vi "Do_ADAM_channel.vi"(4 "Scan Period":dbl format="%.2f", 5 "Previous Scan Value":dbl format="%.2f", 6 "Present scan array":dbl[](array[numeric]) format="%.2f", 7 "Value to Output":dbl format="%.2f", 8 "Ch Description":T1 {"Duty" format="%016b"; "D" format="%#_5g"; "C" format="%#_5g"; "B" format="%#_5g"; "A" format="%#_5g"}, 9 "Ch names":string[](array[string])) -> (0 "Scan comment":string, 1 "Output":dbl format="%.3f")   [LabVIEW 2016]
uses:
  ADAM Client/Sub VIs/ADAM Controls/Ch_description_ADAM.ctl
  ADAM Client/Sub VIs/ADAM Controls/Module_type_ADAM.ctl
  ADAM Client/Sub VIs/ADAM Controls/Function_ADAM.ctl
  ADAM Client/Sub VIs/ADAM Controls/Channel_State.ctl
  ADAM Client/Sub VIs/ADAM Controls/Calib_type_ADAM.ctl
  ADAM Client/Sub VIs/ADAM Controls/Address.ctl
  ADAM Client/Sub VIs/ADAM Controls/Remember_value_mode.ctl
  ADAM Serial/Instrument drivers/Arduino/ctls_and_globals/Arduino tx msg cluster.ctl
  <vilib>/Utility/error.llb/DialogType.ctl
  Anemometry/Anemometry Sub Vis/Controls/In_Range.ctl
  <vilib>/Analysis/baseanly.llb/Mean (DBL).vi
  ADAM Serial/Instrument drivers/LabJack/T7/T7Examples/MODBUS/T7MOD_Read_UINT16_Register.vi
  ADAM Serial/Instrument drivers/LabJack/T7/T7Examples/MODBUS/T7MOD_Read_UINT32_Register.vi
  ADAM Serial/Instrument drivers/LabJack/T7/T7Examples/MODBUS/T7MOD_Read_INT32_Register.vi
  ADAM Serial/Instrument drivers/LabJack/T7/T7Examples/MODBUS/T7MOD_Read_FLOAT32_Register.vi
  ADAM Serial/Instrument drivers/LabJack/T7/T7Examples/MODBUS/T7MOD_Write_UINT16_Register.vi
  ADAM Serial/Instrument drivers/LabJack/T7/T7Examples/MODBUS/T7MOD_Write_UINT32_Register.vi
  ADAM Serial/Instrument drivers/LabJack/T7/T7Examples/MODBUS/T7MOD_Write_INT32_Register.vi
  ADAM Serial/Instrument drivers/LabJack/T7/T7Examples/MODBUS/T7MOD_Write_FLOAT32_Register.vi
  Anemometry/Anemometry Sub Vis/Globals/Gas_management_global.vi
  ADAM_Global.vi
  Anemometry/Anemometry Sub Vis/Globals/Constants_global.vi
  <vilib>/Analysis/NI_AALBase.lvlib
panel:
  in  "MaxAge(s)":dbl=1.5
  in  "History Length":i32=150
  in  "K_Uni_chilled water":dbl=17.0
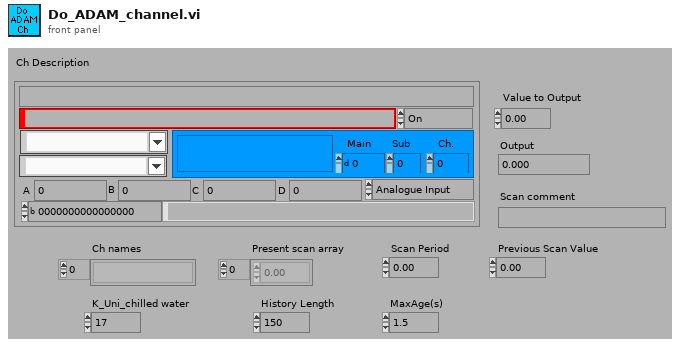
[diagram p1: front panel]
types:
  T1 = typedef "Ch_description_ADAM.ctl" = cluster{"Ch Name":string, "Type":T2, "Function":T3, "Ch State":T4, "Calibration type":T5, "A":dbl, "B":dbl, "C":dbl, "D":dbl, "Comments":string, "Address":T6, "String":string, "Duty":u16}
  T2 = typedef "Module_type_ADAM.ctl" = string
  T3 = typedef "Function_ADAM.ctl" = enum16{"Analogue Input", "Digital Input", "Event counter", "Event rate", "Analogue Output", "Digital Output", "Relay Output"}
  T4 = typedef "Channel_State.ctl" = enum16{"On", "Off", "Always On", "Always Off"}
  T5 = typedef "Calib_type_ADAM.ctl" = string
  T6 = typedef "Address.ctl" = cluster{"Main":i32, "Ch.":i32, "Sub":i32, "Port Name":string}
  T7 = typedef "Remember_value_mode.ctl" = enum16{"Read only", "Read and Write"}
  T8 = cluster{"error out":errorcluster, "source out":string, "message":string, "Read At":timestamp, dbl}
  T9 = cluster{"error out":errorcluster, "source out":string, "message":string}
  T10 = typedef "In_Range.ctl" = enum16{"%", "±", "% & ±"}
  T11 = typedef "Arduino tx msg cluster.ctl" = cluster{"dest":u8, "A/D/C/I":string, "R/W":string, "chan":u8, "val (float)":sgl}
  T12 = typedef "DialogType.ctl" = u16
  T13 = typedef "Valco_valve_ph.ctl" = u16
  T14 = typedef "LVDateTimeRec.ctl" = cluster{"fractional second":dbl, "second":i32, "minute":i32, "hour":i32, "day of month":i32, "month":i32, "year":i32, "day of week":i32, "day of year":i32, "DST":i32}
  T15 = typedef "Client_State_Cluster.ctl" = cluster{"Client Name":string, "Traverse level State":T16, "People to Email":string[], "Next Contact Time":dbl}
  T16 = typedef "Traverse_Level_State.ctl" = enum16{"Running", "Complete"}
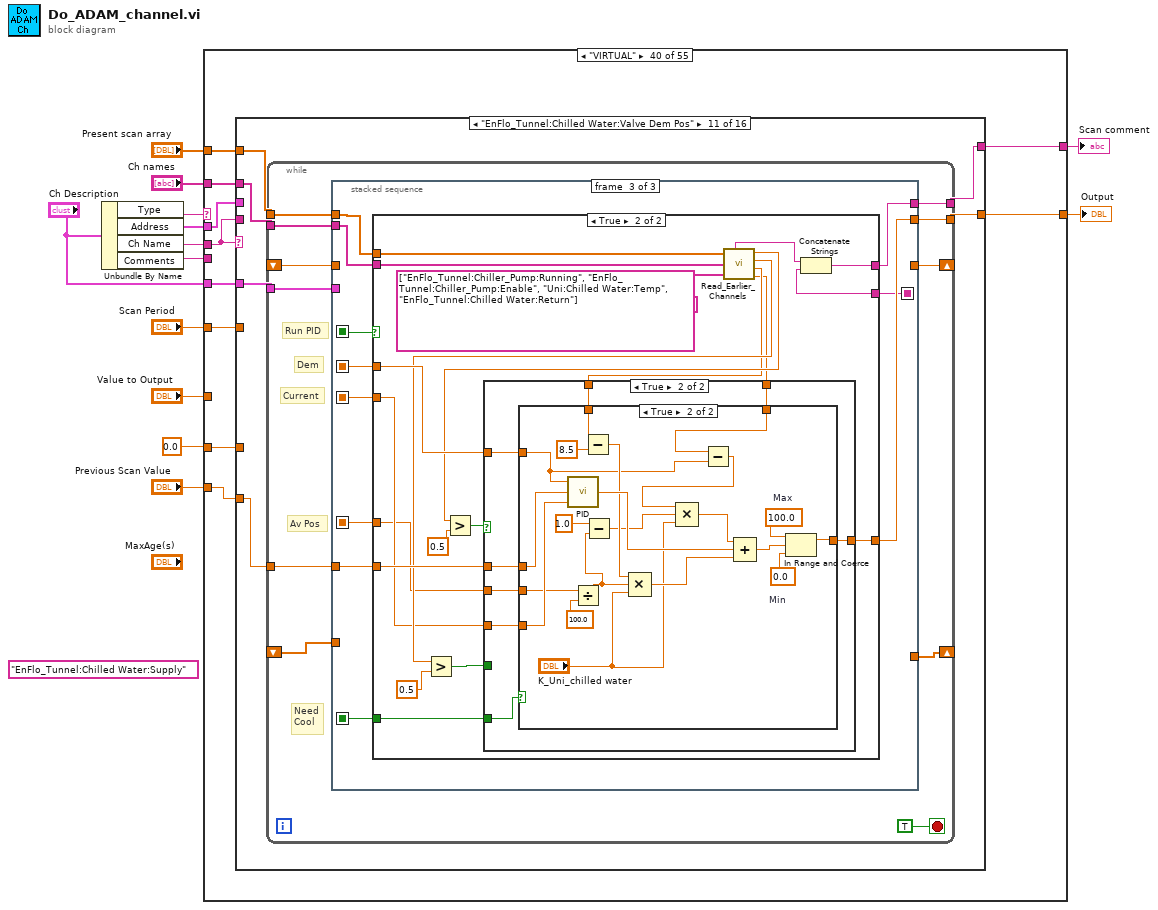
[diagram p0: block diagram]
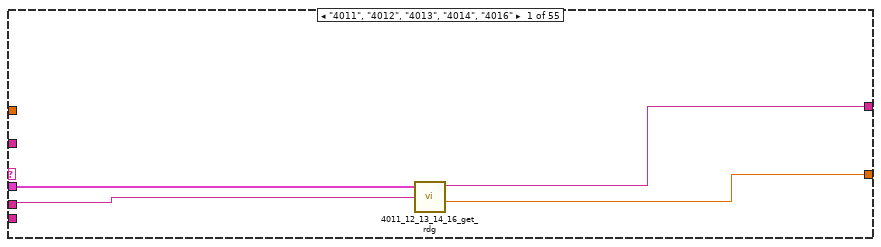
[diagram p2: hidden frame]
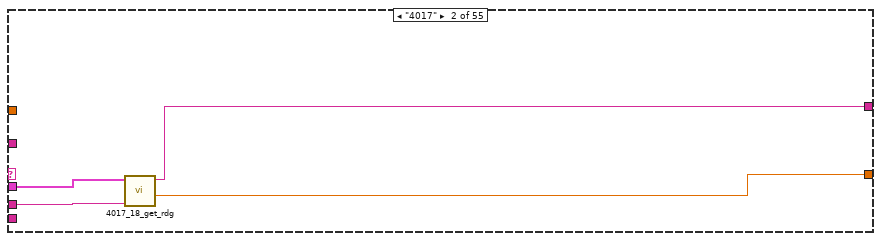
[diagram p3: hidden frame]
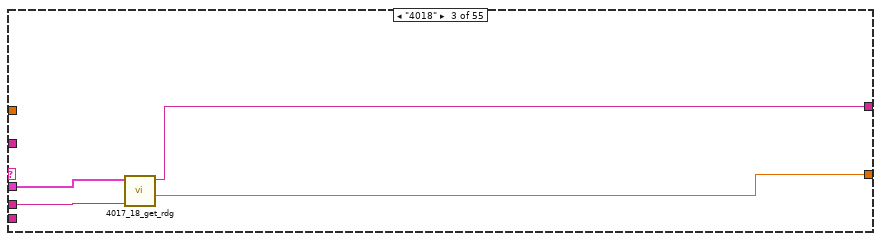
[diagram p4: hidden frame]
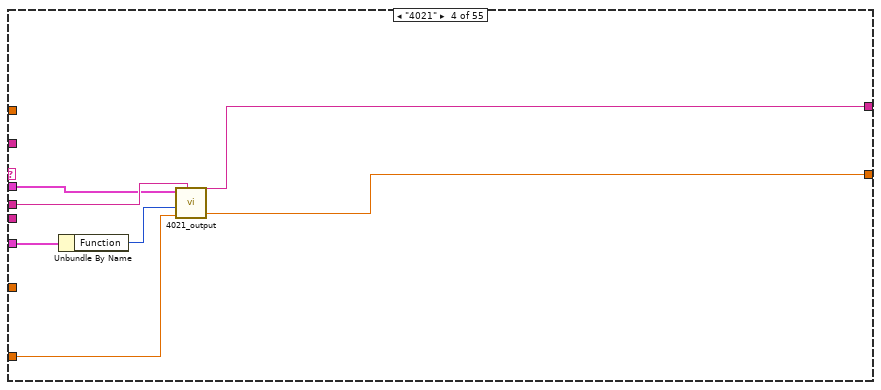
[diagram p5: hidden frame]
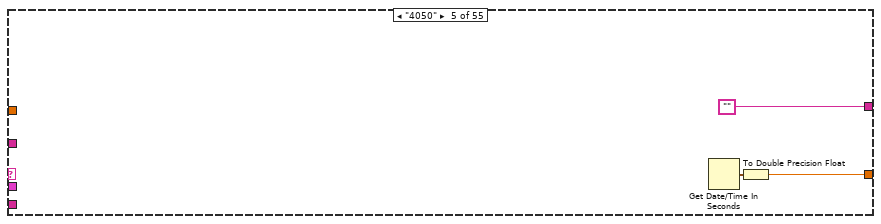
[diagram p6: hidden frame]
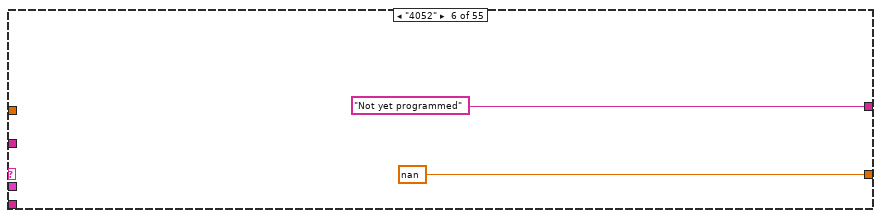
[diagram p7: hidden frame]
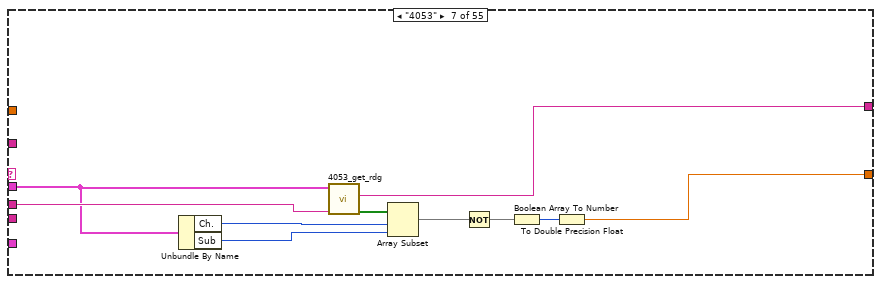
[diagram p8: hidden frame]
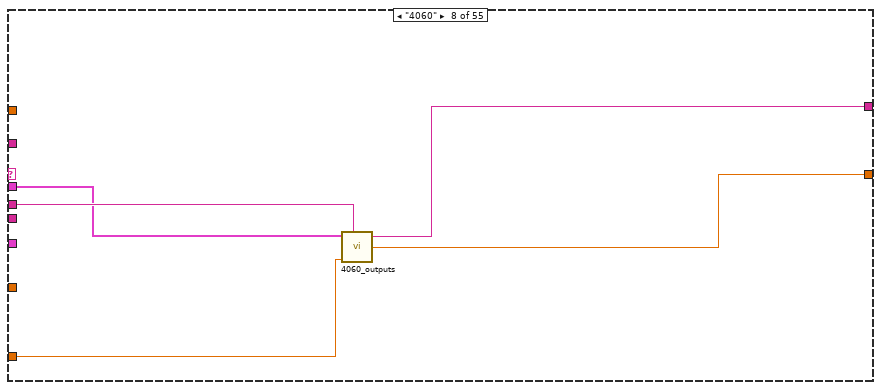
[diagram p9: hidden frame]
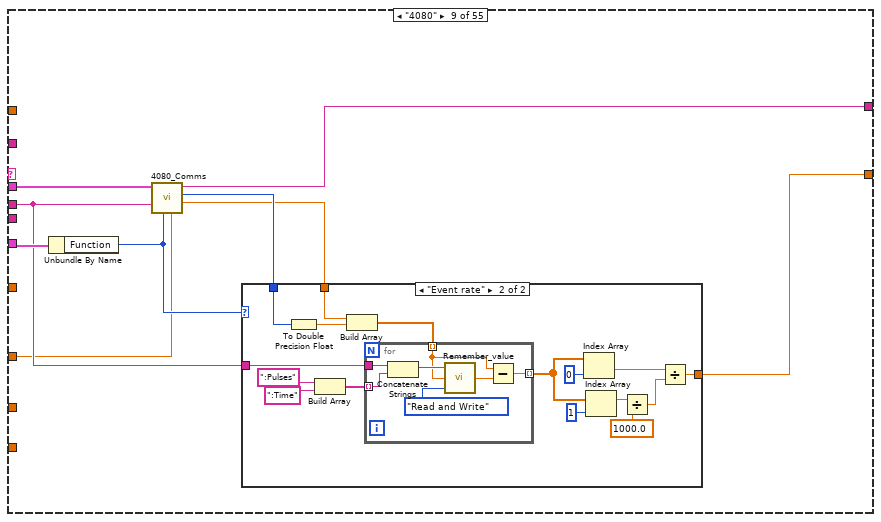
[diagram p10: hidden frame]
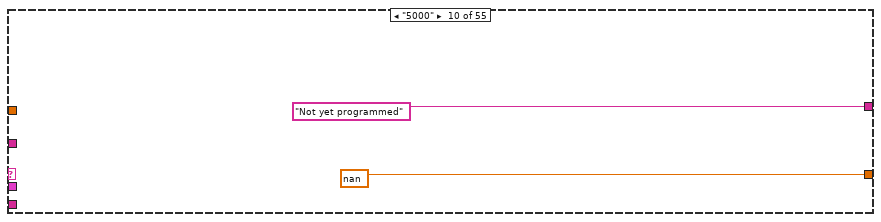
[diagram p12: hidden frame]
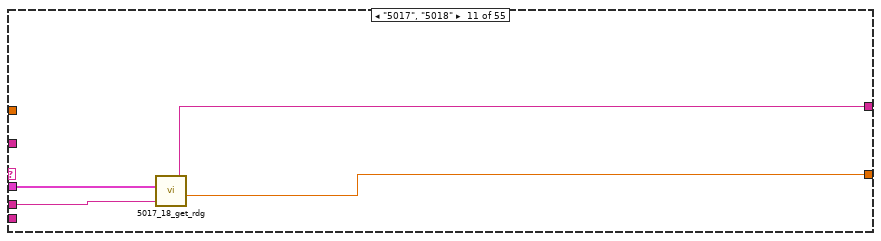
[diagram p13: hidden frame]
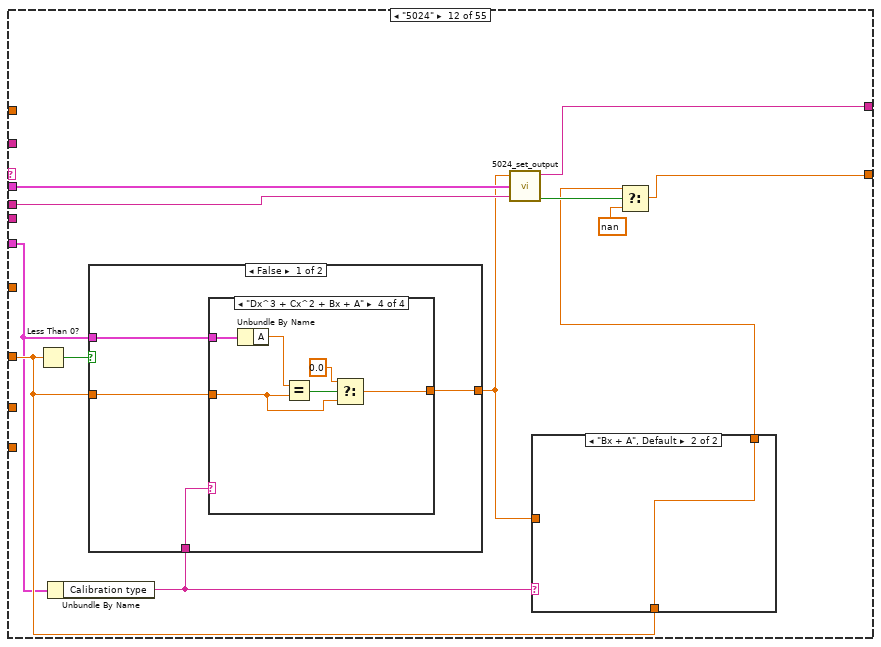
[diagram p14: hidden frame]
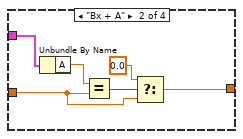
[diagram p17: hidden frame]
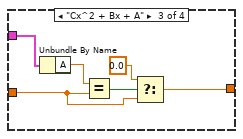
[diagram p18: hidden frame]
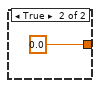
[diagram p19: hidden frame]
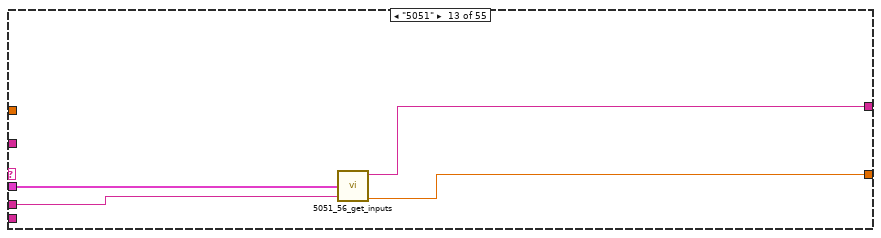
[diagram p20: hidden frame]
diagram:
  (unwired) "EnFlo_Tunnel:Chilled Water:Supply"
  n1 = Unbundle By Name("Ch Description") -> ("Type"=w1:T2, "Address"=w11:T6, "Ch Name"=w3:string, "Comments"=w8:string)
  n2 = case shown="\"VIRTUAL\"" w1 {
    tunnel: [w16 w20 w24 w31 w34 nan w41 w50 w59 nan w89 w99 w131 w139 w160 w182 w201 w216 w232 w261 w281 w380 w492 nan w499 w501 w508 w510 w526 w539 w868 w1127 w1134 w1135 w1141 w1204 w1222 nan w1263 w1282 w1880 w1888 w1893 w1905 w1919 w1924 w1931 w1934 w1939 w1945 w1950 w1974 w1997 w2026 0.0 ("Output")] -> w9
    tunnel: [w17 w21 w25 w32 "" "Not yet programmed" w46 w51 w61 "Not yet programmed" w90 w102 w132 w138 w161 w183 w200 w219 w234 w256 w280 w379 w493 "Not yet programmed" w498 w502 w507 w511 w525 w538 w869 w1128 w1133 w1139 w1143 w1205 w1214 "Not yet programmed" "" w1281 w1881 w1887 "" "" w1918 w1925 "" w1935 "" w1944 "" "Crazy time based random number!" w1986 w2025 "Warning; unmatched case in Do_ADAM_channel" ("Status note")] -> w6
    tunnel: w11 -> [w14 w18 w22 w26 _ _ w38 w49 w53 _ w91 w103 w133 w137 w162 w184 w215 w231 w247 w272 w285 w384 w491 _ _ _ w505 w509 w528 _ _ w1130 w1131 w1137 w1145 w1210 w1219 _ w1272 w1273 _ _ _ _ _ _ _ _ _ _ _ _ _ _ _]
    tunnel: "Ch Description" -> [_ _ _ w30 _ _ _ _ w60 _ _ w92 _ w136 w159 w181 _ _ _ _ _ _ _ _ w500 w504 _ _ _ w540 w871 _ _ _ w1144 _ _ _ _ w1275 w1885 w1892 _ _ w1921 w1929 _ w1936 w1940 w1946 _ _ _ w2031 _]
    tunnel: w3 -> [w15 w19 w23 w27 _ _ w47 w52 w56 _ w88 w98 w130 w134 w156 w178 _ _ _ _ _ _ _ _ _ _ w506 _ w527 _ _ w1129 w1132 w1138 w1142 w1209 w1215 _ _ w1278 _ _ _ w1901 _ _ _ _ _ _ _ _ w1993 _ _]
    tunnel: "Ch names" -> [_ _ _ _ _ _ _ _ _ _ _ _ _ _ _ _ _ _ _ _ _ _ _ _ _ _ _ _ _ _ _ _ _ _ _ _ _ _ _ w1280 w1886 w1891 _ _ w1922 w1930 _ w1937 _ _ _ _ _ w2032 _]
    tunnel: "Present scan array" -> [_ _ _ _ _ _ _ _ _ _ _ _ _ _ _ _ _ _ _ _ _ _ _ _ _ _ _ _ _ _ _ _ _ _ _ _ _ _ _ w1279 w1884 w1889 _ _ w1920 w1928 _ w1938 _ _ _ _ _ w2029 _]
    tunnel: w8 -> [_ _ _ _ _ _ _ _ _ _ _ _ _ _ _ _ _ _ _ _ _ _ _ _ _ _ _ _ _ _ _ _ _ _ _ _ _ _ _ _ _ _ _ _ _ _ _ _ _ _ _ _ _ w2024 _]
    tunnel: "Value to Output" -> [_ _ _ w28 _ _ _ w48 w54 _ _ w94 _ w135 w157 w179 _ w217 w233 _ _ _ _ _ w497 w503 _ _ w524 w541 w870 _ _ _ w1140 _ w1223 _ w1267 _ w1882 _ _ _ _ w1926 _ _ _ _ _ _ _ w2030 _]
    tunnel: "Scan Period" -> [_ _ _ _ _ _ _ _ _ _ _ _ _ _ _ _ _ _ _ _ _ _ _ _ _ _ _ _ _ _ _ _ _ _ _ _ _ _ _ w1277 w1883 w1890 _ _ _ w1927 _ _ _ w1942 w1951 _ _ w2027 _]
    tunnel: "Previous Scan Value" -> [_ _ _ _ _ _ _ _ _ _ _ _ _ _ _ _ w203 _ _ w248 w279 w378 _ _ w496 _ _ _ _ _ _ _ _ _ _ _ _ _ _ w1276 w1879 _ w1893 _ w1917 w1923 w1931 _ _ w1943 w1948 _ _ w2028 _]
    tunnel: 0.0 -> [_ _ _ _ _ _ _ _ _ _ _ _ _ _ _ _ _ _ _ _ _ _ _ _ _ _ _ _ _ _ _ _ _ _ _ _ _ _ _ w1274 _ _ _ _ _ _ _ _ _ _ _ _ _ _ _]
    frame "4011", "4012", "4013", "4014", "4016" {
      n3 = call "4011_12_13_14_16_get_rdg.vi"("Address"=w14, "Channel Name"=w15) -> ("Comment"=w17:string, "Reading"=w16:dbl)  [unwired: 1 in, 2 out]
    }
    frame "4017" {
      n4 = call "4017_18_get_rdg.vi"("Channel Name"=w19, "Address"=w18) -> ("Reading"=w20:dbl, "Comment"=w21:string)  [unwired: 2 in, 2 out]
    }
    frame "4018" {
      n5 = call "4017_18_get_rdg.vi"("Channel Name"=w23, "Address"=w22) -> ("Reading"=w24:dbl, "Comment"=w25:string)  [unwired: 2 in, 2 out]
    }
    frame "4021" {
      n6 = Unbundle By Name(w30) -> ("Function"=w29:T3)
      n7 = call "4021_output.vi"("Address"=w26, "Function"=w29, "Set to:"=w28, "Channel Name"=w27) -> ("Comment"=w32:string, "Reading"=w31:dbl)  [unwired: 1 in, 1 out]
    }
    frame "4050" {
      n8 = Get Date/Time In Seconds() -> (seconds since 1Jan1904=w33:timestamp)
      n9 = To Double Precision Float(number=w33) -> (double precision float=w34:dbl)
    }
    frame "4052" {
    }
    frame "4053" {
      n10 = Unbundle By Name(w38) -> ("Ch."=w39:i32, "Sub"=w45:i32)
      n11 = call "4053_get_rdg.vi"("Channel Name"=w47, "Address"=w38) -> ("Boolean array"=w44:bool[], "Comment"=w46:string)  [unwired: 2 in, 2 out]
      n12 = Array Subset(array=w44, index=w39, length=w45) -> (w43:bool[])
      n13 = Not(x=w43) -> (.not. x?=w40:bool[])
      n14 = Boolean Array To Number(Boolean array=w40) -> (number=w42:u32)
      n15 = To Double Precision Float(number=w42) -> (double precision float=w41:dbl)
    }
    frame "4060" {
      n16 = call "4060_outputs.vi"("Address"=w49, "Value to Output"=w48, "Channel Name"=w52) -> ("Comment"=w51:string, "Reading"=w50:dbl)  [unwired: 2 in, 1 out]
    }
    frame "4080" {
      n17 = Unbundle By Name(w60) -> ("Function"=w55:T3)
      n18 = call "4080_Comms.vi"("Value to display"=w54, "Function"=w55, "Channel Name"=w56, "Address"=w53) -> ("Reading"=w57:dbl, "millisecond timer value"=w58:u32, "Comment"=w61:string)  [unwired: 2 in, 1 out]
      n19 = case shown="\"Event rate\"" w55 {
        tunnel: w56 -> [_ w78]
        tunnel: w58 -> [_ w71]
        tunnel: [w62 w63] -> w59
        tunnel: w57 -> [w62 w72]
        frame "Event counter", Default {
        }
        frame "Event rate" {
          n20 = To Double Precision Float(number=w71) -> (double precision float=w70:dbl)
          n21 = Build Array(":Pulses", ":Time") -> (w73:string[])
          n22 = Build Array(w72, w70) -> (w69:dbl[])
          n23 = for {
            tunnel: w78 -> [w82]
            tunnel: [w83] -> w66 mode=indexing
            tunnel: w73 -> [w80] mode=indexing
            tunnel: w69 -> [w79] mode=indexing
            n24 = Concatenate Strings(w82, w80) -> (w81:string)
            n25 = call "Remember_value.vi"("Mode"=Remember_value_mode."Read and Write", "Input Value"=w79, "Ch name"=w81) -> ("Output Value"=w84:dbl)
            n26 = Subtract(x=w79, y=w84) -> (x-y=w83:dbl)
          }
          n27 = Index Array(array=w66, index=0) -> (element=w64:dbl)
          n28 = Index Array(array=w66, index=1) -> (element=w65:dbl)
          n29 = Divide(x=w65, y=1000.0) -> (x/y=w76:dbl)
          n30 = Divide(x=w64, y=w76) -> (x/y=w63:dbl)
        }
      }
    }
    frame "5000" {
    }
    frame "5017", "5018" {
      n31 = call "5017_18_get_rdg.vi"("Address (all reqd.)"=w91, "Channel Name"=w88) -> ("Comment"=w90:string, "Reading"=w89:dbl)  [unwired: 3 out]
    }
    frame "5024" {
      n32 = Less Than 0?(x=w94) -> (x < 0?=w97:bool)
      n33 = Unbundle By Name(w92) -> ("Calibration type"=w93:T5)
      n34 = case shown="False" w97 {
        tunnel: [w109 0.0 ("t")] -> w95
        tunnel: w94 -> [w107 _]
        tunnel: w93 -> [w108 _]
        tunnel: w92 -> [w106 _]
        frame False {
          n35 = case shown="\"Dx^3 + Cx^2 + Bx + A\"" w108 {
            tunnel: w107 -> [w110 w113 w119 w125]
            tunnel: w106 -> [_ w116 w122 w128]
            tunnel: [w110 w111 w117 w123] -> w109
            frame "Raw", Default {
            }
            frame "Bx + A" {
              n36 = Unbundle By Name(w116) -> ("A"=w115:dbl)
              n37 = Equal?(x=w115, y=w113) -> (x = y?=w114:bool)
              n38 = Select(t=0.0, s=w114, f=w113) -> (s? t:f=w111:dbl)
            }
            frame "Cx^2 + Bx + A" {
              n39 = Unbundle By Name(w122) -> ("A"=w121:dbl)
              n40 = Equal?(x=w121, y=w119) -> (x = y?=w120:bool)
              n41 = Select(t=0.0, s=w120, f=w119) -> (s? t:f=w117:dbl)
            }
            frame "Dx^3 + Cx^2 + Bx + A" {
              n42 = Unbundle By Name(w128) -> ("A"=w127:dbl)
              n43 = Equal?(x=w127, y=w125) -> (x = y?=w126:bool)
              n44 = Select(t=0.0, s=w126, f=w125) -> (s? t:f=w123:dbl)
            }
          }
        }
        frame True {
        }
      }
      n45 = call "5024_set_output.vi"("Set to:"=w95, "Address (all reqd.)"=w103, "Channel Name"=w98) -> ("Comment"=w102:string, "Good Reply"=w100:bool)  [unwired: 2 out]
      n46 = case shown="\"Bx + A\", Default" w93 {
        tunnel: [w104 w105] -> w96
        tunnel: w95 -> [w104 _]
        tunnel: w94 -> [_ w105]
        frame "Raw" {
        }
        frame "Bx + A", Default {
        }
      }
      n47 = Select(t=w96, s=w100, f=nan) -> (s? t:f=w99:dbl)
    }
    frame "5051" {
      n48 = call "5051_56_get_inputs.vi"("Address (Main, Sub reqd.)"=w133, "Channel Name"=w130) -> ("Comment"=w132:string, "Single output"=w131:dbl)  [unwired: 3 out]
    }
    frame "5056" {
      n49 = Unbundle By Name(w136) -> ("Function"=w140:T3)
      n50 = case shown="\"Relay Output\"" w140 {
        tunnel: w137 -> [_ w146 w155]
        tunnel: ["This function is not available" w147 w153] -> w138
        tunnel: [nan ("A") w144 w150] -> w139
        tunnel: w135 -> [_ _ w149]
        tunnel: w134 -> [_ w143 w148]
        frame "Analogue Input", Default {
        }
        frame "Digital Input" {
          # "Readback value"
          n51 = call "5060_check_outputs.vi"("Address (Main, Sub reqd.)"=w146, "Channel Name"=w143) -> ("Comment"=w147:string, "Single Channel"=w145:i16)  [unwired: 3 out]
          n52 = To Double Precision Float(number=w145) -> (double precision float=w144:dbl)
        }
        frame "Relay Output" {
          # "Sets single o/p channel"
          n53 = Greater Than 0?(x=w149) -> (x > 0?=w154:bool)
          n54 = call "5056_60_set_single_output.vi"("Channel Name"=w148, "Address (all reqd.)"=w155, "Set state:"=w154) -> ("Comment"=w153:string, "Good Reply"=w152:bool)  [unwired: 2 out]
          n55 = Select(t=w149, s=w152, f=nan) -> (s? t:f=w150:dbl)
        }
      }
    }
    frame "5060" {
      n56 = Unbundle By Name(w159) -> ("Function"=w158:T3)
      n57 = case shown="\"Relay Output\"" w158 {
        tunnel: w162 -> [_ w168 w177]
        tunnel: ["This function is not available" w169 w175] -> w161
        tunnel: [nan ("A") w166 w172] -> w160
        tunnel: w157 -> [_ _ w171]
        tunnel: w156 -> [_ w165 w170]
        frame "Analogue Input", Default {
        }
        frame "Digital Input" {
          # "Readback value"
          n58 = call "5060_check_outputs.vi"("Address (Main, Sub reqd.)"=w168, "Channel Name"=w165) -> ("Comment"=w169:string, "Single Channel"=w167:i16)  [unwired: 3 out]
          n59 = To Double Precision Float(number=w167) -> (double precision float=w166:dbl)
        }
        frame "Relay Output" {
          # "Sets single o/p channel"
          n60 = Greater Than 0?(x=w171) -> (x > 0?=w176:bool)
          n61 = call "5056_60_set_single_output.vi"("Channel Name"=w170, "Address (all reqd.)"=w177, "Set state:"=w176) -> ("Comment"=w175:string, "Good Reply"=w174:bool)  [unwired: 2 out]
          n62 = Select(t=w171, s=w174, f=nan) -> (s? t:f=w172:dbl)
        }
      }
    }
    frame "6060" {
      n63 = Unbundle By Name(w181) -> ("Function"=w180:T3)
      n64 = case shown="\"Relay Output\"" w180 {
        tunnel: w184 -> [_ w190 w199]
        tunnel: ["This function is not available" w191 w197] -> w183
        tunnel: [nan ("A") w188 w194] -> w182
        tunnel: w179 -> [_ _ w193]
        tunnel: w178 -> [_ w187 w192]
        frame "Analogue Input", Default {
        }
        frame "Digital Input" {
          n65 = call "6060_read_all_I-O.vi"("Address (Main, Sub reqd.)"=w190, "Channel Name"=w187) -> ("Comment"=w191:string, "Single Input Channel"=w189:i16)  [unwired: 3 out]
          n66 = To Double Precision Float(number=w189) -> (double precision float=w188:dbl)
        }
        frame "Relay Output" {
          # "Sets single o/p channel"
          n67 = Greater Than 0?(x=w193) -> (x > 0?=w198:bool)
          n68 = call "6060_set_single_output.vi"("Channel Name"=w192, "Address (Main, Ch requd.)"=w199, "Set state:"=w198) -> ("Comment"=w197:string, "Good Reply"=w196:bool)  [unwired: 2 out]
          n69 = Select(t=w193, s=w196, f=nan) -> (s? t:f=w194:dbl)
        }
      }
    }
    frame "Arduino A_in" {
      w209 = T11 {"dest"=1, "A/D/C/I"="A", "R/W"="R", "chan"=1, "val (float)"=0.0}  # Tx msg cluster
      # "Analogue read case"
      n70 = Unbundle By Name(w215) -> ("Port Name"=w206:string, "Main"=w207:i32, "Ch."=w208:i32)
      n71 = To Unsigned Byte Integer(number=w207) -> (unsigned 8bit integer=w214:u8)
      n72 = To Unsigned Byte Integer(number=w208) -> (unsigned 8bit integer=w212:u8)
      n73 = Bundle By Name(cluster=w209, "dest"=w214, "A/D/C/I"="A" ("A/D"), "R/W"="R", "chan"=w212, "val (float)"=sgl 0.0) -> (w205:T11)
      n74 = call "Arduino generic wrapper.vi"("Tx msg cluster"=w205, "Port name"=w206) -> ("Scan comment"=w200:string, "Output"=w202:dbl)
      n75 = Empty String/Path?(string/path=w200) -> (empty?=w204:bool)
      n76 = Select(t=w202, s=w204, f=w203) -> (s? t:f=w201:dbl)
    }
    frame "Arduino A_out" {
      w226 = T11 {"dest"=1, "A/D/C/I"="A", "R/W"="R", "chan"=1, "val (float)"=0.0}  # Tx msg cluster
      # "Analogue write case"
      n77 = Unbundle By Name(w231) -> ("Port Name"=w223:string, "Main"=w224:i32, "Ch."=w225:i32)
      n78 = To Unsigned Byte Integer(number=w224) -> (unsigned 8bit integer=w230:u8)
      n79 = To Unsigned Byte Integer(number=w225) -> (unsigned 8bit integer=w229:u8)
      n80 = To Single Precision Float(number=w217) -> (single precision float=w221:sgl)
      n81 = Bundle By Name(cluster=w226, "dest"=w230, "A/D/C/I"="A" ("A/D"), "R/W"="W", "chan"=w229, "val (float)"=w221) -> (w222:T11)
      n82 = call "Arduino generic wrapper.vi"("Tx msg cluster"=w222, "Port name"=w223) -> ("Scan comment"=w219:string)  [unwired: 1 out]
      n83 = Empty String/Path?(string/path=w219) -> (empty?=w218:bool)
      n84 = Select(t=w217, s=w218, f=nan ("Reading")) -> (s? t:f=w216:dbl)
    }
    frame "Arduino D_out" {
      w242 = T11 {"dest"=1, "A/D/C/I"="A", "R/W"="R", "chan"=1, "val (float)"=0.0}  # Tx msg cluster
      # "Digital write case"
      n85 = Unbundle By Name(w247) -> ("Port Name"=w239:string, "Main"=w240:i32, "Ch."=w241:i32)
      n86 = To Unsigned Byte Integer(number=w240) -> (unsigned 8bit integer=w246:u8)
      n87 = To Unsigned Byte Integer(number=w241) -> (unsigned 8bit integer=w245:u8)
      n88 = To Single Precision Float(number=w233) -> (single precision float=w237:sgl)
      n89 = Bundle By Name(cluster=w242, "dest"=w246, "A/D/C/I"="D" ("A/D"), "R/W"="W", "chan"=w245, "val (float)"=w237) -> (w238:T11)
      n90 = call "Arduino generic wrapper.vi"("Tx msg cluster"=w238, "Port name"=w239) -> ("Scan comment"=w234:string)  [unwired: 1 out]
      n91 = Empty String/Path?(string/path=w234) -> (empty?=w235:bool)
      n92 = Select(t=w233, s=w235, f=nan ("Reading")) -> (s? t:f=w232:dbl)
    }
    frame "Arduino Thermistor" {
      w266 = T11 {"dest"=1, "A/D/C/I"="A", "R/W"="R", "chan"=1, "val (float)"=0.0}  # Tx msg cluster
      # "Thermistor read case"
      # "values not expected in 'normal' operating conditions"
      n93 = Unbundle By Name(w272) -> ("Port Name"=w263:string, "Main"=w264:i32, "Ch."=w265:i32)
      n94 = To Unsigned Byte Integer(number=w264) -> (unsigned 8bit integer=w271:u8)
      n95 = To Unsigned Byte Integer(number=w265) -> (unsigned 8bit integer=w269:u8)
      n96 = Bundle By Name(cluster=w266, "dest"=w271, "A/D/C/I"="A" ("A/D"), "R/W"="R", "chan"=w269, "val (float)"=sgl 0.0) -> (w262:T11)
      n97 = call "Arduino generic wrapper.vi"("Tx msg cluster"=w262, "Port name"=w263) -> ("Scan comment"=w252:string, "Output"=w250:dbl)
      n98 = Empty String/Path?(string/path=w252) -> (empty?=w251:bool)
      n99 = Select(t=w250, s=w251, f=w248) -> (s? t:f=w249:dbl)
      n100 = Less?(x=w250, y=-40.0) -> (x < y?=w253:bool)
      n101 = Greater?(x=w250, y=140.0) -> (0:w254:bool)
      n102 = case shown="False" w253 {
        tunnel: [w274 "Faulty thermistor open-circuit;"] -> w255
        tunnel: w254 -> [w273 _]
        frame False {
          n103 = case shown="True" w273 {
            tunnel: ["" "Faulty thermistor short-circuit;"] -> w274
            frame False {
            }
            frame True {
            }
          }
        }
        frame True {
        }
      }
      n104 = Or(x=w253, y=w254) -> (x .or. y?=w258:bool)
      n105 = Select(t=nan ("f"), s=w258, f=w249) -> (s? t:f=w261:dbl)
      n106 = Concatenate Strings(w252, w255) -> (w256:string)
    }
    frame "NaMCU" {
      # "See \"Default\" tab for channel matrix"
      # "PN's \"NaMCU\" devices. Low range pressure transducer with on-board correction, environmental sensor, 2x thermistors, Ain + Aout (5V), Din + Dout"
      n107 = Unbundle By Name(w285) -> ("Port Name"=w282:string, "Main"=w283:i32, "Sub"=w278:i32, "Ch."=w284:i32)
      n108 = case shown="Default" w278 {
        tunnel: w284 -> [w294 w318 w338 w353 w368 _]
        tunnel: w283 -> [w293 w317 w337 w352 w367 _]
        tunnel: w282 -> [w292 w316 w336 w351 w366 _]
        tunnel: [w286 w314 w330 w345 w360 0.0 ("Output")] -> w281
        tunnel: [w287 w309 w332 w347 w362 "Warning; invalid Sub being addressed on a NaMCU device in Do_ADAM_channel.vi"] -> w280
        tunnel: w279 -> [w288 w301 w333 w348 w363 _]
        frame 0 {
          w295 = T11 {"dest"=1, "A/D/C/I"="A", "R/W"="R", "chan"=1, "val (float)"=0.0}  # Tx msg cluster
          # "Get pressure (Pa)"
          n109 = To Unsigned Byte Integer(number=w293) -> (unsigned 8bit integer=w300:u8)
          n110 = To Unsigned Byte Integer(number=w294) -> (unsigned 8bit integer=w298:u8)
          n111 = Bundle By Name(cluster=w295, "dest"=w300, "A/D/C/I"="P" ("A/D"), "R/W"="R", "chan"=w298, "val (float)"=sgl 0.0) -> (w291:T11)
          n112 = call "Arduino generic wrapper.vi"("Tx msg cluster"=w291, "Port name"=w292) -> ("Scan comment"=w287:string, "Output"=w289:dbl)
          n113 = Empty String/Path?(string/path=w287) -> (empty?=w290:bool)
          n114 = Select(t=w289, s=w290, f=w288) -> (s? t:f=w286:dbl)
        }
        frame 1 {
          w319 = T11 {"dest"=1, "A/D/C/I"="A", "R/W"="R", "chan"=1, "val (float)"=0.0}  # Tx msg cluster
          # "values not expected in 'normal' operating conditions"
          # "Get temperature (deg C)"
          n115 = To Unsigned Byte Integer(number=w317) -> (unsigned 8bit integer=w324:u8)
          n116 = To Unsigned Byte Integer(number=w318) -> (unsigned 8bit integer=w322:u8)
          n117 = Bundle By Name(cluster=w319, "dest"=w324, "A/D/C/I"="T" ("A/D"), "R/W"="R", "chan"=w322, "val (float)"=sgl 0.0) -> (w315:T11)
          n118 = call "Arduino generic wrapper.vi"("Tx msg cluster"=w315, "Port name"=w316) -> ("Scan comment"=w305:string, "Output"=w303:dbl)
          n119 = Empty String/Path?(string/path=w305) -> (empty?=w304:bool)
          n120 = Select(t=w303, s=w304, f=w301) -> (s? t:f=w302:dbl)
          n121 = Less?(x=w303, y=-40.0) -> (x < y?=w306:bool)
          n122 = Greater?(x=w303, y=140.0) -> (0:w307:bool)
          n123 = case shown="False" w306 {
            tunnel: [w326 "Faulty thermistor open-circuit;"] -> w308
            tunnel: w307 -> [w325 _]
            frame False {
              n124 = case shown="True" w325 {
                tunnel: ["" "Faulty thermistor short-circuit;"] -> w326
                frame False {
                }
                frame True {
                }
              }
            }
            frame True {
            }
          }
          n125 = Or(x=w306, y=w307) -> (x .or. y?=w311:bool)
          n126 = Select(t=nan ("f"), s=w311, f=w302) -> (s? t:f=w314:dbl)
          n127 = Concatenate Strings(w305, w308) -> (w309:string)
        }
        frame 2 {
          w339 = T11 {"dest"=1, "A/D/C/I"="A", "R/W"="R", "chan"=1, "val (float)"=0.0}  # Tx msg cluster
          # "Get relative humidity (%)"
          n128 = To Unsigned Byte Integer(number=w337) -> (unsigned 8bit integer=w344:u8)
          n129 = To Unsigned Byte Integer(number=w338) -> (unsigned 8bit integer=w342:u8)
          n130 = Bundle By Name(cluster=w339, "dest"=w344, "A/D/C/I"="H" ("A/D"), "R/W"="R", "chan"=w342, "val (float)"=sgl 0.0) -> (w335:T11)
          n131 = call "Arduino generic wrapper.vi"("Tx msg cluster"=w335, "Port name"=w336) -> ("Scan comment"=w332:string, "Output"=w331:dbl)
          n132 = Empty String/Path?(string/path=w332) -> (empty?=w334:bool)
          n133 = Select(t=w331, s=w334, f=w333) -> (s? t:f=w330:dbl)
        }
        frame 3 {
          w354 = T11 {"dest"=1, "A/D/C/I"="A", "R/W"="R", "chan"=1, "val (float)"=0.0}  # Tx msg cluster
          # "Get fluid density (kg/m^3)"
          n134 = To Unsigned Byte Integer(number=w352) -> (unsigned 8bit integer=w359:u8)
          n135 = To Unsigned Byte Integer(number=w353) -> (unsigned 8bit integer=w357:u8)
          n136 = Bundle By Name(cluster=w354, "dest"=w359, "A/D/C/I"="R" ("A/D"), "R/W"="R", "chan"=w357, "val (float)"=sgl 0.0) -> (w350:T11)
          n137 = call "Arduino generic wrapper.vi"("Tx msg cluster"=w350, "Port name"=w351) -> ("Scan comment"=w347:string, "Output"=w346:dbl)
          n138 = Empty String/Path?(string/path=w347) -> (empty?=w349:bool)
          n139 = Select(t=w346, s=w349, f=w348) -> (s? t:f=w345:dbl)
        }
        frame 4 {
          w369 = T11 {"dest"=1, "A/D/C/I"="A", "R/W"="R", "chan"=1, "val (float)"=0.0}  # Tx msg cluster
          # "Get flow speed (pitot-static equivalent) (m/s)"
          n140 = To Unsigned Byte Integer(number=w367) -> (unsigned 8bit integer=w374:u8)
          n141 = To Unsigned Byte Integer(number=w368) -> (unsigned 8bit integer=w372:u8)
          n142 = Bundle By Name(cluster=w369, "dest"=w374, "A/D/C/I"="U" ("A/D"), "R/W"="R", "chan"=w372, "val (float)"=sgl 0.0) -> (w365:T11)
          n143 = call "Arduino generic wrapper.vi"("Tx msg cluster"=w365, "Port name"=w366) -> ("Scan comment"=w362:string, "Output"=w361:dbl)
          n144 = Empty String/Path?(string/path=w362) -> (empty?=w364:bool)
          n145 = Select(t=w361, s=w364, f=w363) -> (s? t:f=w360:dbl)
        }
        frame Default {
          # "dP_sensor and flow speed are time-averaged between calls"
          # "Oh dear, user has created a server channel with an invalid \"sub\" address"
        }
      }
    }
    frame "NaCTA" {
      # "See \"Default\" tab for channel matrix"
      # "PN's \"NaCTA\" devices. Thermistor CTA with on-board calibration drift compensation, environmental sensor, 6-axis IMU."
      n146 = Unbundle By Name(w384) -> ("Port Name"=w381:string, "Main"=w382:i32, "Sub"=w377:i32, "Ch."=w383:i32)
      n147 = case shown="Default" w377 {
        tunnel: w383 -> [w393 w417 w437 w452 w467 w482 _]
        tunnel: w382 -> [w392 w416 w436 w451 w466 w481 _]
        tunnel: w381 -> [w391 w415 w435 w450 w465 w480 _]
        tunnel: [w385 w413 w429 w444 w459 w474 0.0 ("Output")] -> w380
        tunnel: [w386 w408 w431 w446 w461 w476 "Warning; invalid Sub being addressed on a NaCTA device in Do_ADAM_channel.vi"] -> w379
        tunnel: w378 -> [w387 w400 w432 w447 w462 w477 _]
        frame 0 {
          w394 = T11 {"dest"=1, "A/D/C/I"="A", "R/W"="R", "chan"=1, "val (float)"=0.0}  # Tx msg cluster
          # "Get atmospheric pressure (Pa)"
          n148 = To Unsigned Byte Integer(number=w392) -> (unsigned 8bit integer=w399:u8)
          n149 = To Unsigned Byte Integer(number=w393) -> (unsigned 8bit integer=w397:u8)
          n150 = Bundle By Name(cluster=w394, "dest"=w399, "A/D/C/I"="P" ("A/D"), "R/W"="R", "chan"=w397, "val (float)"=sgl 0.0) -> (w390:T11)
          n151 = call "Arduino generic wrapper.vi"("Tx msg cluster"=w390, "Port name"=w391) -> ("Scan comment"=w386:string, "Output"=w388:dbl)
          n152 = Empty String/Path?(string/path=w386) -> (empty?=w389:bool)
          n153 = Select(t=w388, s=w389, f=w387) -> (s? t:f=w385:dbl)
        }
        frame 1 {
          w418 = T11 {"dest"=1, "A/D/C/I"="A", "R/W"="R", "chan"=1, "val (float)"=0.0}  # Tx msg cluster
          # "values not expected in 'normal' operating conditions"
          # "Get temperature (deg C)"
          n154 = To Unsigned Byte Integer(number=w416) -> (unsigned 8bit integer=w423:u8)
          n155 = To Unsigned Byte Integer(number=w417) -> (unsigned 8bit integer=w421:u8)
          n156 = Bundle By Name(cluster=w418, "dest"=w423, "A/D/C/I"="T" ("A/D"), "R/W"="R", "chan"=w421, "val (float)"=sgl 0.0) -> (w414:T11)
          n157 = call "Arduino generic wrapper.vi"("Tx msg cluster"=w414, "Port name"=w415) -> ("Scan comment"=w404:string, "Output"=w402:dbl)
          n158 = Empty String/Path?(string/path=w404) -> (empty?=w403:bool)
          n159 = Select(t=w402, s=w403, f=w400) -> (s? t:f=w401:dbl)
          n160 = Less?(x=w402, y=-40.0) -> (x < y?=w405:bool)
          n161 = Greater?(x=w402, y=140.0) -> (0:w406:bool)
          n162 = case shown="False" w405 {
            tunnel: [w425 "Faulty thermistor open-circuit;"] -> w407
            tunnel: w406 -> [w424 _]
            frame False {
              n163 = case shown="True" w424 {
                tunnel: ["" "Faulty thermistor short-circuit;"] -> w425
                frame False {
                }
                frame True {
                }
              }
            }
            frame True {
            }
          }
          n164 = Or(x=w405, y=w406) -> (x .or. y?=w410:bool)
          n165 = Select(t=nan ("f"), s=w410, f=w401) -> (s? t:f=w413:dbl)
          n166 = Concatenate Strings(w404, w407) -> (w408:string)
        }
        frame 2 {
          w438 = T11 {"dest"=1, "A/D/C/I"="A", "R/W"="R", "chan"=1, "val (float)"=0.0}  # Tx msg cluster
          # "Get relative humidity (%)"
          n167 = To Unsigned Byte Integer(number=w436) -> (unsigned 8bit integer=w443:u8)
          n168 = To Unsigned Byte Integer(number=w437) -> (unsigned 8bit integer=w441:u8)
          n169 = Bundle By Name(cluster=w438, "dest"=w443, "A/D/C/I"="H" ("A/D"), "R/W"="R", "chan"=w441, "val (float)"=sgl 0.0) -> (w434:T11)
          n170 = call "Arduino generic wrapper.vi"("Tx msg cluster"=w434, "Port name"=w435) -> ("Scan comment"=w431:string, "Output"=w430:dbl)
          n171 = Empty String/Path?(string/path=w431) -> (empty?=w433:bool)
          n172 = Select(t=w430, s=w433, f=w432) -> (s? t:f=w429:dbl)
        }
        frame 3 {
          w453 = T11 {"dest"=1, "A/D/C/I"="A", "R/W"="R", "chan"=1, "val (float)"=0.0}  # Tx msg cluster
          # "Get fluid property"
          n173 = To Unsigned Byte Integer(number=w451) -> (unsigned 8bit integer=w458:u8)
          n174 = To Unsigned Byte Integer(number=w452) -> (unsigned 8bit integer=w456:u8)
          n175 = Bundle By Name(cluster=w453, "dest"=w458, "A/D/C/I"="R" ("A/D"), "R/W"="R", "chan"=w456, "val (float)"=sgl 0.0) -> (w449:T11)
          n176 = call "Arduino generic wrapper.vi"("Tx msg cluster"=w449, "Port name"=w450) -> ("Scan comment"=w446:string, "Output"=w445:dbl)
          n177 = Empty String/Path?(string/path=w446) -> (empty?=w448:bool)
          n178 = Select(t=w445, s=w448, f=w447) -> (s? t:f=w444:dbl)
        }
        frame 4 {
          w468 = T11 {"dest"=1, "A/D/C/I"="A", "R/W"="R", "chan"=1, "val (float)"=0.0}  # Tx msg cluster
          # "Get flow speed (m/s). Time-averaged between calls."
          n179 = To Unsigned Byte Integer(number=w466) -> (unsigned 8bit integer=w473:u8)
          n180 = To Unsigned Byte Integer(number=w467) -> (unsigned 8bit integer=w471:u8)
          n181 = Bundle By Name(cluster=w468, "dest"=w473, "A/D/C/I"="U" ("A/D"), "R/W"="R", "chan"=w471, "val (float)"=sgl 0.0) -> (w464:T11)
          n182 = call "Arduino generic wrapper.vi"("Tx msg cluster"=w464, "Port name"=w465) -> ("Scan comment"=w461:string, "Output"=w460:dbl)
          n183 = Empty String/Path?(string/path=w461) -> (empty?=w463:bool)
          n184 = Select(t=w460, s=w463, f=w462) -> (s? t:f=w459:dbl)
        }
        frame 5 {
          w483 = T11 {"dest"=1, "A/D/C/I"="A", "R/W"="R", "chan"=1, "val (float)"=0.0}  # Tx msg cluster
          # "Get IMU value"
          n185 = To Unsigned Byte Integer(number=w481) -> (unsigned 8bit integer=w488:u8)
          n186 = To Unsigned Byte Integer(number=w482) -> (unsigned 8bit integer=w486:u8)
          n187 = Bundle By Name(cluster=w483, "dest"=w488, "A/D/C/I"="X" ("A/D"), "R/W"="R", "chan"=w486, "val (float)"=sgl 0.0) -> (w479:T11)
          n188 = call "Arduino generic wrapper.vi"("Tx msg cluster"=w479, "Port name"=w480) -> ("Scan comment"=w476:string, "Output"=w475:dbl)
          n189 = Empty String/Path?(string/path=w476) -> (empty?=w478:bool)
          n190 = Select(t=w475, s=w478, f=w477) -> (s? t:f=w474:dbl)
        }
        frame Default {
          # "N.B. all fluid properties (sub 3) are evaluated at T_film"
          # "Oh dear, user has created a server channel with an invalid \"sub\" address"
        }
      }
    }
    frame "ClimatronicsUDP" {
      # "Climatronics sonic anemometer thru Serial to Ether converter"
      n191 = call "ClimatronicsUDP_get_rdg.vi"("Address"=w491) -> ("Output"=w492:dbl, "Status note"=w493:string)  [unwired: 5 in]
    }
    frame "DRUCK" {
    }
    frame "DLI WebPowerSwitch" {
      # "https://www.digital-loggers.com/lpc.html"
      n192 = call "DLIWebPowerSwitch.vi"("Previous Scan Value"=w496, "Value to Output"=w497, "Ch Description"=w500) -> ("Scan comment"=w498:string, "Output"=w499:dbl)  [unwired: 4 in, 1 out]
    }
    frame "AalborgMFC" {
      n193 = call "AalborgMFC.vi"("Value to Output"=w503, "Ch Description"=w504) -> ("Scan comment"=w502:string, "Output"=w501:dbl)  [unwired: 5 in, 1 out]
    }
    frame "GILL" {
      n194 = call "Gill_get_rdg.vi"("Channel Name"=w506, "Address"=w505) -> ("Output"=w508:dbl, "Status note"=w507:string)  [unwired: 2 in, 2 out]
    }
    frame "IR2100" {
      n195 = call "IR2100_get_rdg.vi"("Address"=w509) -> ("Comment"=w511:string, "Reading"=w510:dbl)  [unwired: 2 in, 2 out]
    }
    frame "JEM" {
      n196 = Unbundle By Name(w528) -> ("Main"=w514:i32, "Ch."=w513:i32, "Port Name"=w523:string)
      n197 = case shown="0, Default" w513 {
        tunnel: [i16[] [-3, -2, -1, 0, 14, 29, 43, 57, 71, 86, 100] i16[] [0, 20, 40, 60, 80, 100, 120]] -> w517
        tunnel: [u8[] [10, 50, 80, 100, 120, 140, 160, 180, 200, 220, 240] u8[] [20, 50, 90, 130, 160, 200, 230]] -> w518
        frame 0, Default {
        }
        frame 1 {
        }
      }
      n198 = Add(x=w514, y=w513) -> (x+y=w512:i32)
      n199 = Threshold 1D Array(2:w524, 3:w517) -> (0:w520:dbl)  [unwired: 1 out]
      n200 = Round To Nearest(number=w520) -> (nearest integer value=w521:dbl)
      n201 = To Long Integer(number=w521) -> (32bit integer=w519:i32)
      n202 = Index Array(array=w518, index=w519) -> (element=w516:u8)
      n203 = call "DMX.vi"("Port Name"=w523, "DMX channel no."=w512, "Set value:"=w516, "Channel Name"=w527) -> ("error"=w522:bool)  [unwired: 2 out]
      n204 = Index Array(array=w517, index=w519) -> (element=w515:i16)
      n205 = case shown="False" w522 {
        tunnel: [w529 nan] -> w526
        tunnel: ["" "Comms Error"] -> w525
        tunnel: w515 -> [w531 _]
        frame False {
          n206 = To Double Precision Float(number=w531) -> (double precision float=w529:dbl)
        }
        frame True {
        }
      }
    }
    frame "LabJack T7" {
      # "Type : LabJack T7 is used to read & write high level IO. The T7 has AIN#(0:14), AOUT#(0:1), DIO#(0:22)"
      n207 = Unbundle By Name(w540) -> ("Function"=w542:T3)
      n208 = case shown="\"Analogue Output\"" w542 {
        tunnel: w540 -> [w545 w629 w707 w791]
        tunnel: [w544 w627 w706 w788] -> w538
        tunnel: [w543 w626 w705 w789] -> w539
        tunnel: w541 -> [_ w628 _ w790]
        frame "Analogue Input", Default {
          n209 = while {
            shift-right: [w547] -> _
            shift-left: "CheckAge" -> [w552]
            tunnel: w545 -> [w551]
            tunnel: [w548] -> w544
            tunnel: [w549] -> w543
            stop <- w550 continue-if-true
            n210 = case shown="\"GetValue\"" w552 {
              tunnel: ["" "" w598] -> w548
              tunnel: [w559 w576 w592] -> w547
              tunnel: [TRUE w575 w591] -> w550
              tunnel: [nan w577 w590] -> w549
              tunnel: w551 -> [w555 w573 w589]
              frame "CheckAge", Default {
                # "If the LastRead of a particular T7 occured within the interval specified by the parameter MaxAge [seconds], then the stored value will be returned; otherwise, a \"fresher\" value will be acquired."
                n211 = Unbundle By Name(w555) -> ("Address.Port Name"=w554:string)
                n212 = Concatenate Strings(w554, "LastRead" ("string")) -> (w569:string)
                n213 = call "Remember_value.vi"("Mode"=Remember_value_mode."Read only", "Ch name"=w569) -> ("Output Value"=w564:dbl)  [unwired: 1 in]
                n214 = Get Date/Time In Seconds() -> (seconds since 1Jan1904=w566:timestamp)
                n215 = local read "MaxAge(s)"() -> (w553:dbl)
                n216 = To Double Precision Float(number=w566) -> (double precision float=w565:dbl)
                n217 = Subtract(x=w565, y=w564) -> (x-y=w563:dbl)
                n218 = Less Or Equal?(x=w563, y=w553) -> (x <= y?=w562:bool)
                n219 = Select(t="GetValue", s=w562, f="ReadRegisters") -> (s? t:f=w559:string)
              }
              frame "GetValue" {
                # "An acceptably \"fresh\" value is available, so it is read from shift register in Remember_value.vi and returned to Output"
                n220 = Unbundle By Name(w573) -> ("Address.Port Name"=w571:string, "Address.Ch."=w570:i32)
                n221 = Format Into String(format string="(%d)", initial string=w571, w570) -> (resulting string=w574:string)  [unwired: 1 in, 1 out]
                n222 = call "Remember_value.vi"("Mode"=Remember_value_mode."Read only", "Ch name"=w574) -> ("Output Value"=w577:dbl)  [unwired: 1 in]
                n223 = Not A Number/Path/Refnum?(number/path/refnum=w577) -> (NaN/Path/Refnum?=w575:bool)
                n224 = case shown="True" w575 {
                  tunnel: ["" "ReadRegisters"] -> w576
                  tunnel: w574 -> [w582 _]
                  frame False {
                    # "Once a Channel value is read, ensure that a new value is acquired by writing NaN to shift registerfor that Channel."
                    n225 = call "Remember_value.vi"("Mode"=Remember_value_mode."Read and Write", "Input Value"=nan, "Ch name"=w582) -> ()  [unwired: 1 out]
                  }
                  frame True {
                    # "If the stored value is a NaN, re-ReadRegisters"
                  }
                }
              }
              frame "ReadRegisters" {
                w601 = T12 0 items=["no dialog", "OK message", "continue or stop message", "OK message + warnings", "continue/stop + warnings"] ("type of dialog (OK msg:1)")
                # "For speed, 16 Analog Input Channels are Read at once and stored using shift register in Remember_value.vi. By checking the \"freshness\" of the stored value of each channel, there is no need to read individual channels."
                n226 = Unbundle By Name(w589) -> ("Ch Name"=w586:string, "Address.Port Name"=w587:string, "Address.Main"=w588:i32)
                n227 = call "T7_Read_Float_Registers.vi"("Num Registers"=u16 32, "FirstChannel"=u16 0 ("Starting Address"), "Remote Port"=w588, "Remote IP Address"=w587) -> ("error out"=w597:errorcluster, "ReadAt"=w593:timestamp, "Array"=w594:dbl[])  [unwired: 4 in, 1 out]
                n228 = call <vilib>:"Simple Error Handler.vi"("error source (\" \")"=w586, "type of dialog (OK msg:1)"=w601, "error in (no error)"=w597) -> ("source out"=w599:string, "error out"=w585:errorcluster, "message"=w600:string)  [unwired: 4 out]
                n229 = case shown="No Error" w585 {
                  tunnel: w600 -> [_ w623]
                  tunnel: w599 -> [_ w624]
                  tunnel: ["" w622] -> w598
                  tunnel: w594 -> [w608 _]
                  tunnel: w593 -> [w607 _]
                  tunnel: ["GetValue" "CheckAge"] -> w592
                  tunnel: [TRUE FALSE] -> w591
                  tunnel: [nan nan] -> w590
                  tunnel: w587 -> [w602 _]
                  frame No Error {
                    # "Store Read time and Values in shift register"
                    n230 = for {
                      tunnel: w608 -> [w618] mode=indexing
                      tunnel: w602 -> [w613]
                      i -> [w614]
                      # "Store the N (16) values associated with a particular T7 in shift register"
                      n231 = Format Into String(format string="(%d)", initial string=w613, w614) -> (resulting string=w617:string)  [unwired: 1 in, 1 out]
                      n232 = call "Remember_value.vi"("Mode"=Remember_value_mode."Read and Write", "Input Value"=w618, "Ch name"=w617) -> ()  [unwired: 1 out]
                    }
                    n233 = Concatenate Strings(w602, "LastRead" ("string")) -> (w611:string)
                    n234 = To Double Precision Float(number=w607) -> (double precision float=w606:dbl)
                    n235 = call "Remember_value.vi"("Mode"=Remember_value_mode."Read and Write", "Input Value"=w606, "Ch name"=w611) -> ()  [unwired: 1 out]
                  }
                  frame Error {
                    # "Return Error and Escape While Loop"
                    n236 = Concatenate Strings(w624, w623) -> (w622:string)
                  }
                }
              }
            }
          }
        }
        frame "Analogue Output" {
          n237 = while {
            tunnel: w629 -> [w636]
            tunnel: [w634] -> w627
            tunnel: w628 -> [w635]
            tunnel: [w633] -> w626
            shift-right: [w632] -> _
            shift-left: "CompareDemands" -> [w630]
            stop <- w631 continue-if-true
            n238 = case shown="\"SetValue\"" w630 {
              tunnel: w636 -> [w645 w669 w693]
              tunnel: w635 -> [w637 w655 w694]
              tunnel: [w638 w668 w686] -> w634
              tunnel: [w637 w664 w684] -> w633
              tunnel: [w639 w663 _] -> w632
              tunnel: [w640 w662 FALSE] -> w631
              frame "CompareDemands", Default {
                n239 = Unbundle By Name(w645) -> ("Address.Port Name"=w644:string, "Address.Ch."=w643:i32)  [unwired: 1 out]
                n240 = Format Into String(format string="(DAC%d)", initial string=w644, w643) -> (resulting string=w648:string)  [unwired: 1 in, 1 out]
                n241 = call "Remember_value.vi"("Mode"=Remember_value_mode."Read only", "Ch name"=w648) -> ("Output Value"=w642:dbl)  [unwired: 1 in]
                n242 = Not Equal?(x=w642, y=w637) -> (x != y?=w641:bool)
                n243 = case shown="False" w641 {
                  tunnel: [FALSE TRUE] -> w640
                  tunnel: ["CompareDemands" "SetValue"] -> w639
                  tunnel: ["" ""] -> w638
                  frame False {
                  }
                  frame True {
                  }
                }
              }
              frame "SetValue" {
                w660 = T12 0 items=["no dialog", "OK message", "continue or stop message", "OK message + warnings", "continue/stop + warnings"] ("type of dialog (OK msg:1)")
                n244 = Unbundle By Name(w669) -> ("Ch Name"=w665:string, "Address.Port Name"=w667:string, "Address.Main"=w666:i32, "Address.Ch."=w656:i32)
                n245 = call "T7_Write_Float_Register.vi"("Remote IP Address"=w667, "Remote Port"=w666, "FirstChannel"=w656, "FLOAT32 to Write"=w655) -> ("error out"=w661:errorcluster)  [unwired: 5 in, 1 out]
                n246 = call <vilib>:"Simple Error Handler.vi"("error source (\" \")"=w665, "type of dialog (OK msg:1)"=w660, "error in (no error)"=w661) -> ("source out"=w658:string, "error out"=w659:errorcluster, "message"=w657:string)  [unwired: 4 out]
                n247 = case shown="No Error" w659 {
                  tunnel: w658 -> [_ w683]
                  tunnel: w657 -> [_ w682]
                  tunnel: ["" w681] -> w668
                  tunnel: [w670 nan ("Output Value")] -> w664
                  tunnel: w667 -> [w673 _]
                  tunnel: [_ "CompareDemands"] -> w663
                  tunnel: [FALSE FALSE] -> w662
                  tunnel: w656 -> [w671 _]
                  tunnel: w655 -> [w670 _]
                  frame No Error {
                    n248 = Format Into String(format string="(DAC%d)", initial string=w673, w671) -> (resulting string=w676:string)  [unwired: 1 in, 1 out]
                    n249 = call "Remember_value.vi"("Mode"=Remember_value_mode."Read and Write", "Input Value"=w670, "Ch name"=w676) -> ()  [unwired: 1 out]
                  }
                  frame Error {
                    n250 = Concatenate Strings(w683, w682) -> (w681:string)
                  }
                }
              }
              frame "CheckBounds" {
                n251 = Unbundle By Name(w693) -> ("Address.Ch."=w692:i32)
                n252 = In Range and Coerce(upper limit=1, x=w692, lower limit=0) -> (In Range?=w691:bool)  [unwired: 1 out]
                n253 = In Range and Coerce(upper limit=5.0, x=w694, lower limit=0.0) -> (coerced(x)=w685:dbl, In Range?=w690:bool)
                n254 = case shown="False" w691 {
                  tunnel: ["Invalid Channel Number <0,1>" ""] -> w688
                  frame False {
                  }
                  frame True {
                  }
                }
                n255 = case shown="False" w690 {
                  tunnel: ["Invalid Voltage Demand <0,5>" ""] -> w687
                  tunnel: w685 -> [_ w701]
                  tunnel: [nan w701] -> w684
                  frame False {
                  }
                  frame True {
                  }
                }
                n256 = Concatenate Strings(w688, w687) -> (w686:string)
              }
            }
          }
        }
        frame "Digital Input" {
          n257 = while {
            shift-right: [w709] -> _
            shift-left: "CheckAge" -> [w714]
            tunnel: w707 -> [w713]
            tunnel: [w710] -> w706
            tunnel: [w711] -> w705
            stop <- w712 continue-if-true
            n258 = case shown="\"CheckAge\", Default" w714 {
              tunnel: ["" "" w760] -> w710
              tunnel: [w721 w738 w759] -> w709
              tunnel: [TRUE w737 w758] -> w712
              tunnel: [nan w739 w757] -> w711
              tunnel: w713 -> [w717 w735 w756]
              frame "CheckAge", Default {
                # "If the LastRead of a particular T7 occured within the interval specified by the parameter MaxAge [seconds], then the stored value will be returned; otherwise, a \"fresher\" value will be acquired."
                n259 = Unbundle By Name(w717) -> ("Address.Port Name"=w716:string)
                n260 = Concatenate Strings(w716, "DIOLastRead" ("string")) -> (w731:string)
                n261 = call "Remember_value.vi"("Mode"=Remember_value_mode."Read only", "Ch name"=w731) -> ("Output Value"=w726:dbl)  [unwired: 1 in]
                n262 = Get Date/Time In Seconds() -> (seconds since 1Jan1904=w728:timestamp)
                n263 = local read "MaxAge(s)"() -> (w715:dbl)
                n264 = To Double Precision Float(number=w728) -> (double precision float=w727:dbl)
                n265 = Subtract(x=w727, y=w726) -> (x-y=w725:dbl)
                n266 = Less Or Equal?(x=w725, y=w715) -> (x <= y?=w724:bool)
                n267 = Select(t="GetValue", s=w724, f="ReadRegisters") -> (s? t:f=w721:string)
              }
              frame "GetValue" {
                # "An acceptably \"fresh\" value is available, so it is read from shift register in Remember_value.vi and returned to Output"
                n268 = Unbundle By Name(w735) -> ("Address.Port Name"=w733:string, "Address.Ch."=w732:i32)
                n269 = Format Into String(format string="(DI%d)", initial string=w733, w732) -> (resulting string=w736:string)  [unwired: 1 in, 1 out]
                n270 = call "Remember_value.vi"("Mode"=Remember_value_mode."Read only", "Ch name"=w736) -> ("Output Value"=w739:dbl)  [unwired: 1 in]
                n271 = Not A Number/Path/Refnum?(number/path/refnum=w739) -> (NaN/Path/Refnum?=w737:bool)
                n272 = case shown="False" w737 {
                  tunnel: ["" "ReadRegisters"] -> w738
                  tunnel: w736 -> [w744 _]
                  frame False {
                    # "Once a Channel value is read, ensure that a new value is acquired by writing NaN to shift registerfor that Channel."
                    n273 = call "Remember_value.vi"("Mode"=Remember_value_mode."Read and Write", "Input Value"=nan, "Ch name"=w744) -> ()  [unwired: 1 out]
                  }
                  frame True {
                    # "If the stored value is a NaN, re-ReadRegisters"
                  }
                }
              }
              frame "ReadRegisters" {
                w763 = T12 0 items=["no dialog", "OK message", "continue or stop message", "OK message + warnings", "continue/stop + warnings"] ("type of dialog (OK msg:1)")
                # "For speed, 23 Digital Input Channels are Read at once and stored using shift register in Remember_value.vi. By checking the \"freshness\" of the stored value of each channel, there is no need to read individual channels."
                n274 = Unbundle By Name(w756) -> ("Ch Name"=w755:string, "Address.Port Name"=w750:string, "Address.Main"=w751:i32)
                n275 = call "T7_Read_UINT16_Register.vi"("Num Registers to read"=u16 23 ("Num Registers"), "FirstChannel"=u16 0 ("Starting Address"), "Remote Port"=w751, "Remote IP Address"=w750) -> ("error out"=w749:errorcluster, "LastRead"=w748:timestamp, "Raw Data Read"=w747:u16[])  [unwired: 4 in, 1 out]
                n276 = call <vilib>:"Simple Error Handler.vi"("error source (\" \")"=w755, "type of dialog (OK msg:1)"=w763, "error in (no error)"=w749) -> ("source out"=w761:string, "error out"=w754:errorcluster, "message"=w762:string)  [unwired: 4 out]
                n277 = case shown="No Error" w754 {
                  tunnel: w762 -> [_ w785]
                  tunnel: w761 -> [_ w786]
                  tunnel: ["" w784] -> w760
                  tunnel: w747 -> [w770 _]
                  tunnel: w748 -> [w769 _]
                  tunnel: ["GetValue" "CheckAge"] -> w759
                  tunnel: [TRUE FALSE] -> w758
                  tunnel: [nan nan] -> w757
                  tunnel: w750 -> [w764 _]
                  frame No Error {
                    # "Store Read time and Values in shift register"
                    n278 = for {
                      tunnel: w770 -> [w780] mode=indexing
                      tunnel: w764 -> [w775]
                      i -> [w776]
                      # "Store the N (16) values associated with a particular T7 in shift register"
                      n279 = Format Into String(format string="(DI%d)", initial string=w775, w776) -> (resulting string=w779:string)  [unwired: 1 in, 1 out]
                      n280 = call "Remember_value.vi"("Mode"=Remember_value_mode."Read and Write", "Input Value"=w780, "Ch name"=w779) -> ()  [unwired: 1 out]
                    }
                    n281 = Concatenate Strings(w764, "DIOLastRead" ("string")) -> (w773:string)
                    n282 = To Double Precision Float(number=w769) -> (double precision float=w768:dbl)
                    n283 = call "Remember_value.vi"("Mode"=Remember_value_mode."Read and Write", "Input Value"=w768, "Ch name"=w773) -> ()  [unwired: 1 out]
                  }
                  frame Error {
                    # "Return Error and Escape While Loop"
                    n284 = Concatenate Strings(w786, w785) -> (w784:string)
                  }
                }
              }
            }
          }
        }
        frame "Digital Output" {
          n285 = while {
            tunnel: w791 -> [w798]
            tunnel: [w796] -> w788
            tunnel: w790 -> [w797]
            tunnel: [w795] -> w789
            shift-right: [w794] -> _
            shift-left: "CompareDemands" -> [w792]
            stop <- w793 continue-if-true
            n286 = case shown="\"CheckBounds\"" w792 {
              tunnel: w798 -> [w807 w832 w856]
              tunnel: w797 -> [w799 w818 w857]
              tunnel: [w800 w831 w849] -> w796
              tunnel: [w799 w829 w847] -> w795
              tunnel: [w801 w828 _] -> w794
              tunnel: [w802 w827 FALSE] -> w793
              frame "CompareDemands", Default {
                n287 = Unbundle By Name(w807) -> ("Address.Port Name"=w806:string, "Address.Ch."=w805:i32)  [unwired: 1 out]
                n288 = Format Into String(format string="(DO%d)", initial string=w806, w805) -> (resulting string=w810:string)  [unwired: 1 in, 1 out]
                n289 = call "Remember_value.vi"("Mode"=Remember_value_mode."Read only", "Ch name"=w810) -> ("Output Value"=w804:dbl)  [unwired: 1 in]
                n290 = Not Equal?(x=w804, y=w799) -> (x != y?=w803:bool)
                n291 = case shown="True" w803 {
                  tunnel: [FALSE TRUE] -> w802
                  tunnel: ["CompareDemands" "SetValue"] -> w801
                  tunnel: ["" ""] -> w800
                  frame False {
                  }
                  frame True {
                  }
                }
              }
              frame "SetValue" {
                w826 = T12 0 items=["no dialog", "OK message", "continue or stop message", "OK message + warnings", "continue/stop + warnings"] ("type of dialog (OK msg:1)")
                n292 = Unbundle By Name(w832) -> ("Ch Name"=w830:string, "Address.Port Name"=w821:string, "Address.Main"=w822:i32, "Address.Ch."=w820:i32)
                n293 = To Unsigned Word Integer(number=w818) -> (unsigned 16bit integer=w817:u16)
                n294 = call "T7_Write_UINT16_Register.vi"("Remote IP Address"=w821, "Remote Port"=w822, "FirstChannel"=w820, "UINT16 to Write"=w817) -> ("error out"=w819:errorcluster)  [unwired: 5 in, 1 out]
                n295 = call <vilib>:"Simple Error Handler.vi"("error source (\" \")"=w830, "type of dialog (OK msg:1)"=w826, "error in (no error)"=w819) -> ("source out"=w824:string, "error out"=w825:errorcluster, "message"=w823:string)  [unwired: 4 out]
                n296 = case shown="No Error" w825 {
                  tunnel: w824 -> [_ w846]
                  tunnel: w823 -> [_ w845]
                  tunnel: ["" w844] -> w831
                  tunnel: [w833 nan ("Output Value")] -> w829
                  tunnel: w821 -> [w836 _]
                  tunnel: [_ "CompareDemands"] -> w828
                  tunnel: [FALSE FALSE] -> w827
                  tunnel: w820 -> [w834 _]
                  tunnel: w818 -> [w833 _]
                  frame No Error {
                    n297 = Format Into String(format string="(DO%d)", initial string=w836, w834) -> (resulting string=w839:string)  [unwired: 1 in, 1 out]
                    n298 = call "Remember_value.vi"("Mode"=Remember_value_mode."Read and Write", "Input Value"=w833, "Ch name"=w839) -> ()  [unwired: 1 out]
                  }
                  frame Error {
                    n299 = Concatenate Strings(w846, w845) -> (w844:string)
                  }
                }
              }
              frame "CheckBounds" {
                n300 = Unbundle By Name(w856) -> ("Address.Ch."=w855:i32)
                n301 = In Range and Coerce(upper limit=22, x=w855, lower limit=0) -> (In Range?=w854:bool)  [unwired: 1 out]
                n302 = In Range and Coerce(upper limit=1.0, x=w857, lower limit=0.0) -> (coerced(x)=w848:dbl, In Range?=w853:bool)
                n303 = case shown="True" w854 {
                  tunnel: ["Invalid Channel Number <0,22>" ""] -> w851
                  frame False {
                  }
                  frame True {
                  }
                }
                n304 = case shown="True" w853 {
                  tunnel: ["Invalid Digital Demand <0,1>" ""] -> w850
                  tunnel: w848 -> [_ w864]
                  tunnel: [nan w864] -> w847
                  frame False {
                  }
                  frame True {
                  }
                }
                n305 = Concatenate Strings(w851, w850) -> (w849:string)
              }
            }
          }
        }
      }
    }
    frame "LabJack T7 MODBUS" {
      # "Type : LabJack T7 MODBUS  = access to the MODBUS Map registers. Consult T7 Datasheet for target register description."
      n306 = Unbundle By Name(w871) -> ("Function"=w872:T3)
      n307 = case shown="\"Analogue Input\", Default" w872 {
        tunnel: w871 -> [w875 w1019]
        tunnel: [w874 w1017] -> w869
        tunnel: [w873 w1016] -> w868
        tunnel: w870 -> [_ w1018]
        frame "Analogue Input", Default {
          n308 = while {
            shift-right: [w877] -> _
            shift-left: "CheckDataType" -> [w882]
            tunnel: w875 -> [w881]
            tunnel: [w878] -> w874
            tunnel: [w879] -> w873
            stop <- w880 continue-if-true
            n309 = case shown="\"ReadRegisters\"" w882 {
              tunnel: ["" "" "" w960] -> w878
              tunnel: ["CheckAge" w907 w924 w959] -> w877
              tunnel: [TRUE TRUE w923 w958] -> w880
              tunnel: [nan ("Output Value") nan w925 w957] -> w879
              tunnel: w881 -> [w887 w903 w921 w956]
              frame "CheckDataType" {
                # "For now, this should live in the DataType spec should live in the Comments field. If the field is empty or improperly populated, the correct DataType spec will be fetched and updated. This should only happen on the first scan for a given Channel."
                n310 = Unbundle By Name(w887) -> ("Address.Ch."=w892:i32, "Comments"=w889:string)
                n311 = Match First String(2:string[] ["BYTE", "UINT16", "UINT32", "UINT64", "INT32", "FLOAT32", "STRING"] ("Array"), 3:w889) -> (0:w890:i32)  [unwired: 1 out]
                n312 = Less Than 0?(x=w890) -> (x < 0?=w891:bool)
                n313 = case shown="True" w891 {
                  tunnel: w892 -> [_ w897]
                  tunnel: w887 -> [_ w894]
                  frame False {
                  }
                  frame True {
                    n314 = call "ReadLJMconstants.vi"("Selected Register"=w897) -> ("Data Type"=w893:string)  [unwired: 2 out]
                    n315 = Bundle By Name(cluster=w894, "Comments"=w893) -> (w895:T1)
                    n316 = Build Array(w895) -> (w896:T1[])
                    n317 = call "Update_Ch_Discription_client.vi"("Channels to update In"=w896) -> ()  [unwired: 1 out]
                  }
                }
              }
              frame "CheckAge", Default {
                # "If the LastRead of a particular T7 occured within the interval specified by the parameter MaxAge [seconds], then the stored value will be returned; otherwise, a \"fresher\" value will be acquired."
                n318 = Unbundle By Name(w903) -> ("Address.Port Name"=w900:string, "Address.Ch."=w899:i32)
                n319 = Format Into String(format string="(%d)MOD", initial string=w900, w899) -> (resulting string=w898:string)  [unwired: 1 in, 1 out]
                n320 = Concatenate Strings(w898, "LastRead" ("string")) -> (w917:string)
                n321 = call "Remember_value.vi"("Mode"=Remember_value_mode."Read only", "Ch name"=w917) -> ("Output Value"=w912:dbl)  [unwired: 1 in]
                n322 = Get Date/Time In Seconds() -> (seconds since 1Jan1904=w914:timestamp)
                n323 = local read "MaxAge(s)"() -> (w902:dbl)
                n324 = To Double Precision Float(number=w914) -> (double precision float=w913:dbl)
                n325 = Subtract(x=w913, y=w912) -> (x-y=w911:dbl)
                n326 = Less Or Equal?(x=w911, y=w902) -> (x <= y?=w910:bool)
                n327 = Select(t="GetValue", s=w910, f="ReadRegisters") -> (s? t:f=w907:string)
              }
              frame "GetValue" {
                # "An acceptably \"fresh\" value is available, so it is read from shift register in Remember_value.vi and returned to Output"
                n328 = Unbundle By Name(w921) -> ("Address.Port Name"=w919:string, "Address.Ch."=w918:i32)
                n329 = Format Into String(format string="(%d)MOD", initial string=w919, w918) -> (resulting string=w922:string)  [unwired: 1 in, 1 out]
                n330 = call "Remember_value.vi"("Mode"=Remember_value_mode."Read only", "Ch name"=w922) -> ("Output Value"=w925:dbl)  [unwired: 1 in]
                n331 = Not A Number/Path/Refnum?(number/path/refnum=w925) -> (NaN/Path/Refnum?=w923:bool)
                n332 = case shown="False" w923 {
                  tunnel: ["" "ReadRegisters"] -> w924
                  tunnel: w922 -> [w930 _]
                  frame False {
                    # "Once a Channel value is read, ensure that a new value is acquired by writing NaN to shift registerfor that Channel."
                    n333 = call "Remember_value.vi"("Mode"=Remember_value_mode."Read and Write", "Input Value"=nan, "Ch name"=w930) -> ()  [unwired: 1 out]
                  }
                  frame True {
                    # "If the stored value is a NaN, re-ReadRegisters"
                  }
                }
              }
              frame "ReadRegisters" {
                w961 = T12 0 items=["no dialog", "OK message", "continue or stop message", "OK message + warnings", "continue/stop + warnings"] ("type of dialog (OK msg:1)")
                # "Rgister (a.k.a. Channel) values are Read and stored using shift register in Remember_value.vi. TCP coms are limited by MaxAges by checking the \"freshness\" of the stored value."
                n334 = Unbundle By Name(w956) -> ("Comments"=w936:string, "Address.Port Name"=w953:string, "Address.Main"=w935:i32, "Address.Ch."=w933:i32, "Ch Name"=w934:string)
                n335 = case shown="\"UINT32\"" w936 {
                  tunnel: w953 -> [_ w975 w982 w989 w996]
                  tunnel: w935 -> [_ w974 w981 w988 w995]
                  tunnel: w933 -> [_ w973 w980 w987 w994]
                  tunnel: [w968 w972 w979 w986 w993] -> w952
                  tunnel: [w962 w971 w978 w985 w992] -> w944
                  tunnel: [nan w969 w976 w983 w990] -> w943
                  tunnel: w934 -> [w966 _ _ _ _]
                  frame "No Match", Default {
                    n336 = Bundle By Name(cluster=errorcluster {"status"=FALSE, "code"=0, "source"=""} ("error constant"), "status"=TRUE, "code"=999, "source"=w966) -> (w968:errorcluster)
                    n337 = Get Date/Time In Seconds() -> (seconds since 1Jan1904=w962:timestamp)
                  }
                  frame "UINT16" {
                    n338 = call-poly "T7MOD_ReadWrite.vi"("LabJack UINT16 Register"=w973, "Remote Port"=w974, "Remote IP Address"=w975) -> ("error out"=w972:errorcluster, "Read At"=w971:timestamp, "Read UINT16"=w970:u16)  [unwired: 5 in, 1 out]
                    n339 = To Double Precision Float(number=w970) -> (double precision float=w969:dbl)
                  }
                  frame "UINT32" {
                    n340 = call-poly "T7MOD_ReadWrite.vi"("LabJack UINT32 Register"=w980, "Remote Port"=w981, "Remote IP Address"=w982) -> ("error out"=w979:errorcluster, "Read At"=w978:timestamp, "Read UINT32"=w977:u32)  [unwired: 5 in, 1 out]
                    n341 = To Double Precision Float(number=w977) -> (double precision float=w976:dbl)
                  }
                  frame "INT32" {
                    n342 = call-poly "T7MOD_ReadWrite.vi"("LabJack INT32 Register"=w987, "Remote Port"=w988, "Remote IP Address"=w989) -> ("error out"=w986:errorcluster, "Read At"=w985:timestamp, "Read INT32"=w984:i32)  [unwired: 5 in, 1 out]
                    n343 = To Double Precision Float(number=w984) -> (double precision float=w983:dbl)
                  }
                  frame "FLOAT32" {
                    n344 = call-poly "T7MOD_ReadWrite.vi"("LabJack FLOAT32 Register"=w994, "Remote Port"=w995, "Remote IP Address"=w996) -> ("error out"=w993:errorcluster, "Read At"=w992:timestamp, "Read FLOAT32"=w991:sgl)  [unwired: 5 in, 1 out]
                    n345 = To Double Precision Float(number=w991) -> (double precision float=w990:dbl)
                  }
                }
                n346 = Format Into String(format string="(%d)MOD", initial string=w953, w933) -> (resulting string=w954:string)  [unwired: 1 in, 1 out]
                n347 = call <vilib>:"General Error Handler.vi"("[user-defined codes]"=i32[] [999], "[user-defined descriptions]"=string[] ["MODBUS not setup for DataType"], "search ni.com link visible?(T)"=FALSE, "type of dialog (OK msg:1)"=w961, "error in (no error)"=w952) -> ("source out"=w946:string, "message"=w945:string, "error out"=w947:errorcluster)  [unwired: 6 in, 2 out]
                n348 = Bundle(cluster=T8 {"error out"={"status"=FALSE, "code"=0, "source"=""}, "source out"="", "message"="", "Read At"=timestamp(0 s since 1904-01-01), 0.0}, "error out"=w947, "source out"=w946, "message"=w945, "Read At"=w944, w943) -> (w948:T8)
                n349 = Unbundle(w948) -> ("error out"=w941:errorcluster, "source out"=w940:string, "message"=w939:string, "Read At"=w938:timestamp, w937:dbl)
                n350 = case shown="No Error" w941 {
                  tunnel: w939 -> [_ w1013]
                  tunnel: w940 -> [_ w1014]
                  tunnel: ["" w1012] -> w960
                  tunnel: w937 -> [w1004 _]
                  tunnel: w938 -> [w1003 _]
                  tunnel: ["GetValue" "CheckAge"] -> w959
                  tunnel: [TRUE FALSE] -> w958
                  tunnel: [nan nan] -> w957
                  tunnel: w954 -> [w997 _]
                  frame No Error {
                    # "Store Read time and Values in shift register"
                    n351 = To Double Precision Float(number=w1003) -> (double precision float=w1002:dbl)
                    n352 = Concatenate Strings(w997, "LastRead" ("string")) -> (w1007:string)
                    n353 = call "Remember_value.vi"("Mode"=Remember_value_mode."Read and Write", "Input Value"=w1002, "Ch name"=w1007) -> ()  [unwired: 1 out]
                    n354 = call "Remember_value.vi"("Mode"=Remember_value_mode."Read and Write", "Input Value"=w1004, "Ch name"=w997) -> ()  [unwired: 1 out]
                  }
                  frame Error {
                    # "Return Error and Escape While Loop"
                    n355 = Concatenate Strings(w1014, w1013) -> (w1012:string)
                  }
                }
              }
            }
          }
        }
        frame "Analogue Output" {
          n356 = while {
            tunnel: w1019 -> [w1026]
            tunnel: [w1024] -> w1017
            tunnel: w1018 -> [w1025]
            tunnel: [w1023] -> w1016
            shift-right: [w1022] -> _
            shift-left: "CheckDataType" -> [w1020]
            stop <- w1021 continue-if-true
            n357 = case shown="\"CompareDemands\", Default" w1020 {
              tunnel: w1026 -> [w1028 w1050 w1066]
              tunnel: w1025 -> [_ w1042 w1065]
              tunnel: ["" w1043 w1083] -> w1024
              tunnel: [nan ("Output Value") w1042 w1082] -> w1023
              tunnel: ["CompareDemands" w1044 w1081] -> w1022
              tunnel: [TRUE w1045 w1080] -> w1021
              frame "CheckDataType" {
                # "ID which MODBUS command instance to use by using / searching MODBUS Map for Data Type expected at register#(Address.Ch). Store Data Type in Ch Description.Comments"
                n358 = Unbundle By Name(w1028) -> ("Address.Ch."=w1036:i32, "Comments"=w1033:string)
                n359 = Match First String(2:string[] ["BYTE", "UINT16", "UINT32", "UINT64", "INT32", "FLOAT32", "STRING"] ("Array"), 3:w1033) -> (0:w1034:i32)  [unwired: 1 out]
                n360 = Less Than 0?(x=w1034) -> (x < 0?=w1035:bool)
                n361 = case shown="True" w1035 {
                  tunnel: w1036 -> [_ w1041]
                  tunnel: w1028 -> [_ w1038]
                  frame False {
                  }
                  frame True {
                    n362 = call "ReadLJMconstants.vi"("Selected Register"=w1041) -> ("Data Type"=w1037:string)  [unwired: 2 out]
                    n363 = Bundle By Name(cluster=w1038, "Comments"=w1037) -> (w1039:T1)
                    n364 = Build Array(w1039) -> (w1040:T1[])
                    n365 = call "Update_Ch_Discription_client.vi"("Channels to update In"=w1040) -> ()  [unwired: 1 out]
                  }
                }
              }
              frame "CompareDemands", Default {
                n366 = Unbundle By Name(w1050) -> ("Address.Port Name"=w1049:string, "Address.Ch."=w1048:i32)  [unwired: 1 out]
                n367 = Format Into String(format string="(%d)MOD", initial string=w1049, w1048) -> (resulting string=w1053:string)  [unwired: 1 in, 1 out]
                n368 = call "Remember_value.vi"("Mode"=Remember_value_mode."Read only", "Ch name"=w1053) -> ("Output Value"=w1047:dbl)  [unwired: 1 in]
                n369 = Not Equal?(x=w1047, y=w1042) -> (x != y?=w1046:bool)
                n370 = case shown="False" w1046 {
                  tunnel: [FALSE TRUE] -> w1045
                  tunnel: ["CheckDataType" "SetValue"] -> w1044
                  tunnel: ["" ""] -> w1043
                  frame False {
                  }
                  frame True {
                  }
                }
              }
              frame "SetValue" {
                w1079 = T12 0 items=["no dialog", "OK message", "continue or stop message", "OK message + warnings", "continue/stop + warnings"] ("type of dialog (OK msg:1)")
                n371 = Unbundle By Name(w1066) -> ("Comments"=w1069:string, "Address.Port Name"=w1061:string, "Address.Main"=w1068:i32, "Address.Ch."=w1060:i32, "Ch Name"=w1067:string)
                n372 = case shown="\"UINT16\"" w1069 {
                  tunnel: w1061 -> [_ w1094 w1100 w1106 w1112]
                  tunnel: w1068 -> [_ w1093 w1099 w1105 w1111]
                  tunnel: w1060 -> [_ w1092 w1098 w1104 w1110]
                  tunnel: [w1088 w1091 w1097 w1103 w1109] -> w1078
                  tunnel: w1067 -> [w1086 _ _ _ _]
                  tunnel: w1065 -> [_ w1090 w1096 w1101 w1108]
                  frame "No Match", Default {
                    n373 = Bundle By Name(cluster=errorcluster {"status"=FALSE, "code"=0, "source"=""} ("error constant"), "status"=TRUE, "code"=999, "source"=w1086) -> (w1088:errorcluster)
                  }
                  frame "UINT16" {
                    n374 = To Unsigned Word Integer(number=w1090) -> (unsigned 16bit integer=w1089:u16)
                    n375 = call-poly "T7MOD_ReadWrite.vi"("UINT16 to Write"=w1089, "LabJack UINT16 Register"=w1092, "Remote Port"=w1093, "Remote IP Address"=w1094) -> ("error out"=w1091:errorcluster)  [unwired: 5 in, 2 out]
                  }
                  frame "UINT32" {
                    n376 = To Unsigned Long Integer(number=w1096) -> (unsigned 32bit integer=w1095:u32)
                    n377 = call-poly "T7MOD_ReadWrite.vi"("UINT32 to Write"=w1095, "LabJack UINT32 Register"=w1098, "Remote Port"=w1099, "Remote IP Address"=w1100) -> ("error out"=w1097:errorcluster)  [unwired: 6 in, 1 out]
                  }
                  frame "INT32" {
                    n378 = To Long Integer(number=w1101) -> (32bit integer=w1102:i32)
                    n379 = call-poly "T7MOD_ReadWrite.vi"("INT32 to Write"=w1102, "LabJack INT32 Register"=w1104, "Remote Port"=w1105, "Remote IP Address"=w1106) -> ("error out"=w1103:errorcluster)  [unwired: 6 in, 1 out]
                  }
                  frame "FLOAT32" {
                    n380 = To Single Precision Float(number=w1108) -> (single precision float=w1107:sgl)
                    n381 = call-poly "T7MOD_ReadWrite.vi"("FLOAT32 to Write"=w1107, "LabJack FLOAT32 Register"=w1110, "Remote Port"=w1111, "Remote IP Address"=w1112) -> ("error out"=w1109:errorcluster)  [unwired: 6 in, 1 out]
                  }
                }
                n382 = call <vilib>:"General Error Handler.vi"("[user-defined codes]"=i32[] [999], "[user-defined descriptions]"=string[] ["MODBUS not setup for DataType"], "search ni.com link visible?(T)"=FALSE, "type of dialog (OK msg:1)"=w1079, "error in (no error)"=w1078) -> ("source out"=w1072:string, "message"=w1071:string, "error out"=w1073:errorcluster)  [unwired: 6 in, 2 out]
                n383 = Bundle(cluster=T9 {"error out"={"status"=FALSE, "code"=0, "source"=""}, "source out"="", "message"=""}, "error out"=w1073, "source out"=w1072, "message"=w1071) -> (w1074:T9)
                n384 = Unbundle(w1074) -> ("error out"=w1064:errorcluster, "source out"=w1063:string, "message"=w1062:string)
                n385 = case shown="No Error" w1064 {
                  tunnel: w1063 -> [_ w1126]
                  tunnel: w1062 -> [_ w1125]
                  tunnel: ["" w1124] -> w1083
                  tunnel: [w1113 nan ("Output Value")] -> w1082
                  tunnel: w1061 -> [w1116 _]
                  tunnel: [_ "CheckDataType"] -> w1081
                  tunnel: [FALSE FALSE] -> w1080
                  tunnel: w1060 -> [w1114 _]
                  tunnel: w1065 -> [w1113 _]
                  frame No Error {
                    n386 = Format Into String(format string="(%d)MOD", initial string=w1116, w1114) -> (resulting string=w1119:string)  [unwired: 1 in, 1 out]
                    n387 = call "Remember_value.vi"("Mode"=Remember_value_mode."Read and Write", "Input Value"=w1113, "Ch name"=w1119) -> ()  [unwired: 1 out]
                  }
                  frame Error {
                    n388 = Concatenate Strings(w1126, w1125) -> (w1124:string)
                  }
                }
              }
            }
          }
        }
      }
    }
    frame "LPA" {
      # "LPA was, IIRC, a serially-polled weighing platform we rented at Surrey for Athena Scaperdas' project at Atkins to weigh a helicopter with rotor running. \nTo add to the fun, it was RS232, so to make it addressable it was polled through an addressable ADAM 485-232 module"
      n389 = call "LPA400_get_rdg.vi"("Channel Name"=w1129, "Address"=w1130) -> ("Output"=w1127:dbl, "Status note"=w1128:string)  [unwired: 4 out]
    }
    frame "PPT" {
      n390 = call "PPT_get_rdg.vi"("Channel Name"=w1132, "Address"=w1131) -> ("Reading"=w1134:dbl, "Comment"=w1133:string)  [unwired: 2 in, 2 out]
    }
    frame "Thermistor" {
      # "Could be replaced with use of an \"Equation\" channel..."
      n391 = call "4017_18_get_rdg.vi"("Channel Name"=w1138, "Address"=w1137) -> ("Reading"=w1136:dbl, "Comment"=w1139:string)  [unwired: 2 in, 2 out]
      n392 = call "Thermistor volts to temperature.vi"("V2 (V)"=w1136) -> ("Temperature (degC)"=w1135:dbl)
    }
    frame "Tracker" {
      # "Intended as a replacement for Gulton-West Octets. Proved to have insoluble problem with CJC when packed in rack."
      n393 = while {
        tunnel: w1145 -> [w1169]
        tunnel: w1144 -> [w1168]
        tunnel: [w1162] -> w1143
        tunnel: w1142 -> [w1161]
        tunnel: [w1155] -> w1141
        tunnel: w1140 -> [w1154]
        i -> [w1151]
        stop <- w1148 continue-if-true
        n394 = Unbundle By Name(w1168) -> ("Function"=w1167:T3)
        n395 = Unbundle By Name(w1169) -> ("Port Name"=w1166:string, "Ch."=w1157:i32, "Main"=w1165:i32, "Sub"=w1164:i32)
        n396 = case shown="\"Analogue Output\"" w1167 {
          tunnel: [enum16{"Set", "Read"}."Set" ("Set") enum16{"Set", "Read"}."Set" ("Set") enum16{"Set", "Read"}."Set" ("Set") enum16{"Set", "Read"}."Set" ("Set") enum16{"Set", "Read"}."Set" ("Set") enum16{"Set", "Read"}."Read" ("Set") enum16{"Set", "Read"}."Read" ("Set")] -> w1152
          tunnel: [enum16{"Logic", "Analogue"}."Analogue" ("Analogue") enum16{"Logic", "Analogue"}."Logic" ("Analogue") enum16{"Logic", "Analogue"}."Logic" ("Analogue") enum16{"Logic", "Analogue"}."Logic" ("Analogue") enum16{"Logic", "Analogue"}."Logic" ("Analogue") enum16{"Logic", "Analogue"}."Logic" ("Analogue") enum16{"Logic", "Analogue"}."Analogue" ("Analogue")] -> w1163
          frame "Analogue Output" {
          }
          frame "Digital Output" {
          }
          frame "Relay Output" {
          }
          frame "Event rate" {
          }
          frame "Event counter" {
          }
          frame "Digital Input" {
          }
          frame "Analogue Input" {
          }
        }
        n397 = call "TalkTracker.vi"("PORT NAME"=w1166, "Set"=w1152, "Channel Name"=w1161, "Value to set"=w1154, "MODULE ADDRESS"=w1165, "LOCATION"=w1157, "NO. LOCATIONS"=w1164, "Analogue"=w1163) -> ("Response"=w1159:string, "Good Set?"=w1146:bool, "Comment out"=w1162:string)  [unwired: 1 in, 4 out]
        n398 = Match Pattern(string=w1159, regular expression="\r\n") -> (before substring=w1158:string)  [unwired: 4 out]
        n399 = case shown="\"Set\"" w1152 {
          tunnel: w1158 -> [_ w1181]
          tunnel: [w1173 w1180] -> w1156
          tunnel: w1154 -> [w1175 _]
          tunnel: nan ("Reading") -> [w1174 w1179]
          tunnel: [w1172 w1177] -> w1149
          tunnel: [0 ("y") 1 ("y")] -> w1147
          tunnel: w1146 -> [w1170 _]
          frame "Set" {
            n400 = Not(x=w1170) -> (.not. x?=w1172:bool)
            n401 = Select(t=w1175, s=w1170, f=w1174) -> (s? t:f=w1173:dbl)
          }
          frame "Read" {
            n402 = String Length(string=w1181) -> (length=w1183:i32)
            n403 = Fract/Exp String To Number(string=w1181, default (0 dbl)=w1179) -> (offset past number=w1184:i32, number=w1182:dbl)  [unwired: 2 out]
            n404 = Equal?(x=w1183, y=w1184) -> (x = y?=w1178:bool)
            n405 = Not(x=w1178) -> (.not. x?=w1177:bool)
            n406 = Select(t=w1182, s=w1178, f=w1179) -> (s? t:f=w1180:dbl)
          }
        }
        n407 = case shown="283" w1157 {
          tunnel: w1156 -> [w1185 w1188]
          tunnel: [w1185 w1186] -> w1155
          frame 0, Default {
          }
          frame 283 {
            n408 = Equal To 0?(x=w1188) -> (x = 0?=w1189:bool)
            n409 = Select(t=nan ("Reading"), s=w1189, f=w1188) -> (s? t:f=w1186:dbl)
          }
        }
        n410 = Less?(x=w1151, y=w1147) -> (x < y?=w1150:bool)
        n411 = And(x=w1149, y=w1150) -> (x .and. y?=w1148:bool)
      }
    }
    frame "Vaisala" {
      # "Thermo-hygrometer"
      n412 = Unbundle By Name(w1210) -> ("Main"=w1206:i32, "Ch."=w1207:i32, "Port Name"=w1208:string)
      n413 = call "HMP231.vi"("Channel Name"=w1209, "Port Name"=w1208, "Channel"=w1207, "Address"=w1206) -> ("Output"=w1204:dbl, "Status note"=w1205:string)  [unwired: 2 out]
    }
    frame "VICI" {
      # "Rotary selctor valve"
      n414 = To Long Integer(number=w1223) -> (32bit integer=w1218:i32)
      n415 = Unbundle By Name(w1219) -> ("Port Name"=w1221:string, "Ch."=w1220:i32)
      n416 = call "Valco_Valve_Position.vi"("Channel Name"=w1215, "Valve Number"=w1220, "Port Name"=w1221, "Requested Posn."=w1218) -> ("Error Message"=w1213:string, "Achieved Posn."=w1216:T13)  [unwired: 2 out]
      n417 = Empty String/Path?(string/path=w1213) -> ()  [unwired: 1 out]
      n418 = case shown="False" TRUE {
        tunnel: w1219 -> [w1230 _]
        tunnel: w1218 -> [w1229 _]
        tunnel: [w1228 w1260] -> w1217
        tunnel: w1216 -> [_ w1260]
        tunnel: w1215 -> [w1227 _]
        tunnel: [w1226 w1259] -> w1214
        tunnel: w1213 -> [_ w1259]
        tunnel: w1213 -> [w1225 _]
        tunnel: "X10" ("Port Name") -> [w1224 _]
        frame False {
          # "Old code to reboot valve with power cycle using X10"
          n419 = stacked-sequence {
            tunnel: w1230 -> [_ _ _ _ _ w1251]
            tunnel: w1229 -> [_ _ _ _ _ w1247]
            tunnel: [_ _ _ _ _ w1250] -> w1228
            tunnel: w1227 -> [_ _ _ _ _ w1249]
            tunnel: [_ _ _ _ _ w1248] -> w1226
            tunnel: w1225 -> [_ w1236 _ _ _ _]
            tunnel: w1224 -> [w1231 _ _ w1239 _ _]
            frame #0 {
              w1233 = 3 items=["-----", "A", "B", "C", "D", "E", "F", "G", "H", "I", "J", "K", "L", "M", "N", "O", "P"] ("House Code")
              n420 = call "X10control.vi"("Port Name"=w1231, "Power Request (ON)"=FALSE, "House Code"=w1233, "Unit No."=5) -> ()  [unwired: 6 out]
            }
            frame #1 {
              n421 = call "Server_Emails.vi"("Message"=w1236, "Contact All clients?"=TRUE, "Subject"="Powering Down FID Valve" ("Error Type")) -> ()  [unwired: 2 in, 3 out]
            }
            frame #2 {
              n422 = Wait (ms)(milliseconds to wait=u32 20000) -> ()  [unwired: 1 out]
            }
            frame #3 {
              w1241 = 3 items=["-----", "A", "B", "C", "D", "E", "F", "G", "H", "I", "J", "K", "L", "M", "N", "O", "P"] ("House Code")
              n423 = call "X10control.vi"("Port Name"=w1239, "Power Request (ON)"=TRUE, "House Code"=w1241, "Unit No."=5) -> ()  [unwired: 6 out]
            }
            frame #4 {
              n424 = Wait (ms)(milliseconds to wait=u32 5000) -> ()  [unwired: 1 out]
            }
            frame #5 {
              n425 = Build Array(1 ("element"), 2 ("element"), w1247) -> (w1244:i32[])
              n426 = for {
                tunnel: w1251 -> [w1256]
                tunnel: [w1255] -> w1250
                tunnel: w1249 -> [w1254]
                tunnel: [w1253] -> w1248
                tunnel: w1244 -> [w1252] mode=indexing
                n427 = Unbundle By Name(w1256) -> ("Port Name"=w1257:string, "Ch."=w1258:i32)
                n428 = call "Valco_Valve_Position.vi"("Channel Name"=w1254, "Valve Number"=w1258, "Port Name"=w1257, "Requested Posn."=w1252) -> ("Error Message"=w1253:string, "Achieved Posn."=w1255:T13)  [unwired: 2 out]
              }
            }
          }
        }
        frame True {
          # "Assume no problems"
        }
      }
      n429 = To Double Precision Float(number=w1217) -> (double precision float=w1222:dbl)
    }
    frame "WEST" {
      # "Proposed new mini-DIN PID controllers?"
    }
    frame "X10" {
      (unwired) 1 items=["-----", "A", "B", "C", "D", "E", "F", "G", "H", "I", "J", "K", "L", "M", "N", "O", "P"] ("House Code")
      # "X10 powerline-signalling controller"
      n430 = Greater Than 0?(x=w1267) -> (x > 0?=w1266:bool)
      n431 = Unbundle By Name(w1272) -> ("Port Name"=w1269:string, "Main"=w1270:i32, "Ch."=w1271:i32)
      n432 = call "X10control.vi"("Port Name"=w1269, "Power Request (ON)"=w1266, "House Code"=w1270, "Unit No."=w1271) -> ()  [unwired: 6 out]
      n433 = Select(t=1.0, s=w1266, f=0.0) -> (s? t:f=w1263:dbl)
    }
    frame "VIRTUAL" {
      n434 = case shown="\"EnFlo_Tunnel:Chilled Water:Valve Dem Pos\"" w1278 {
        tunnel: [w1292 w1306 w1320 w1342 w1357 w1368 w1382 w1405 w1433 w1517 w1519 w1658 w1682 w1755 w1782 w1802] -> w1282
        tunnel: [w1283 w1312 w1318 w1346 w1351 w1366 w1395 w1414 w1434 w1511 w1518 w1657 w1681 w1754 "" w1803] -> w1281
        tunnel: w1280 -> [w1289 w1314 w1324 w1348 w1353 w1371 w1393 w1416 w1436 w1513 w1521 w1663 w1683 w1759 _ w1805]
        tunnel: w1279 -> [w1290 w1313 w1325 w1347 w1352 w1372 w1394 w1415 w1437 w1512 w1522 w1665 w1684 w1761 _ w1804]
        tunnel: w1278 -> [w1287 _ _ _ _ _ _ _ _ _ _ _ _ _ w1777 _]
        tunnel: w1277 -> [w1288 _ _ _ _ _ _ _ _ _ _ w1655 _ w1753 w1782 w1801]
        tunnel: w1276 -> [w1291 _ _ _ _ _ _ _ _ _ w1520 w1659 _ w1756 _ w1800]
        tunnel: w1275 -> [_ _ w1316 _ _ _ _ _ w1438 _ w1523 _ _ _ _ _]
        tunnel: w1274 -> [_ w1305 _ _ _ w1365 _ _ _ _ _ _ _ _ _ _]
        tunnel: w1273 -> [_ _ _ _ _ _ _ _ _ _ _ _ _ _ _ _]
        frame "GMU:Remaining:", Default {
          n435 = Match Pattern(string=w1287, regular expression="GMU:Remaining:" ("String to match")) -> (match substring=w1285:string)  [unwired: 4 out]
          n436 = Empty String/Path?(string/path=w1285) -> (empty?=w1284:bool)
          n437 = case shown="False" w1284 {
            tunnel: [w1299 nan] -> w1292
            tunnel: w1291 -> [w1298 _]
            tunnel: w1290 -> [w1297 _]
            tunnel: w1289 -> [w1296 _]
            tunnel: w1288 -> [w1295 _]
            tunnel: w1287 -> [w1294 _]
            tunnel: [w1293 w1301] -> w1283
            frame False {
              n438 = call "Update_Rem_gas.vi"("Scan Period (s)"=w1295, "Gas Remaining in"=w1298, "Ch name"=w1294, "Ch names"=w1296, "Present scan array"=w1297) -> ("Gas Remaining out"=w1299:dbl, "Comments"=w1293:string)  [unwired: 1 out]
            }
            frame True {
              n439 = Current VI's Path() -> (path=w1303:path)
              n440 = Path To String(path=w1303) -> (string=w1302:string)
              n441 = Concatenate Strings(" was not matched in ", w1302) -> (w1301:string)
            }
          }
        }
        frame "GMU:Source:Meas Q" {
          n442 = call "Calculate_Release_Flowrates.vi"("Ch names"=w1314, "Units"=enum16{"Q l/min", "M_dot Kg/min"}."Q l/min", "Present scan array"=w1313) -> ("Trace"=w1310:dbl, "Carrier"=w1311:dbl, "Scan comments"=w1312:string)
          n443 = Add(x=w1311, y=w1310) -> (x+y=w1307:dbl)
          n444 = Not Equal To 0?(x=w1307) -> (x != 0?=w1308:bool)
          n445 = Select(t=w1307, s=w1308, f=w1305) -> (s? t:f=w1306:dbl)
        }
        frame "GMU:Detector:Strength" {
          n446 = Unbundle By Name(w1316) -> ("C"=w1315:dbl)
          n447 = call "Read_value_of_earlier_Ch.vi"("Desired Ch to Read"="GMU:Detector:Meas Current", "Ch names"=w1324, "Present scan array"=w1325) -> ("Value"=w1321:dbl, "Scan comment"=w1319:string)  [unwired: 1 in]
          n448 = Greater?(x=w1321, y=w1315) -> (0:w1322:bool)
          n449 = case shown="True" w1322 {
            tunnel: w1316 -> [_ w1337]
            tunnel: w1321 -> [_ w1332]
            tunnel: [100.0 ("Eng Values") w1330] -> w1320
            tunnel: ["Fault" w1333] -> w1317
            frame False {
            }
            frame True {
              n450 = Unbundle By Name(w1337) -> ("D"=w1328:dbl, "A"=w1336:dbl, "B"=w1335:dbl)
              n451 = Less?(x=w1332, y=w1328) -> (x < y?=w1331:bool)
              n452 = Build Array(w1336, w1335) -> (w1334:dbl[])
              n453 = call "Polynomial_convert.vi"("Calib constants"=w1334, "Voltage"=w1332) -> ("Eng Values"=w1329:dbl)  [unwired: 4 out]
              n454 = case shown="True" w1331 {
                tunnel: ["Saturated" ""] -> w1333
                tunnel: [100.0 ("Eng Values") w1340] -> w1330
                tunnel: w1329 -> [_ w1340]
                frame False {
                }
                frame True {
                }
              }
            }
          }
          n455 = Concatenate Strings(w1319, w1317) -> (w1318:string)
        }
        frame "GMU:Source:Meas M_dot" {
          n456 = call "Calculate_Release_Flowrates.vi"("Ch names"=w1348, "Units"=enum16{"Q l/min", "M_dot Kg/min"}."M_dot Kg/min", "Present scan array"=w1347) -> ("Trace"=w1344:dbl, "Carrier"=w1345:dbl, "Scan comments"=w1346:string)
          n457 = Add(x=w1345, y=w1344) -> (x+y=w1342:dbl)
        }
        frame "GMU:Source:Meas Density" {
          n458 = Build Array("GMU:Source:Meas M_dot", "GMU:Source:Meas Q") -> (w1354:string[])
          n459 = call "Read_Earlier_Channels.vi"("Present scan array"=w1352, "Ch names"=w1353, "Desired Channels"=w1354) -> ("Scan comments"=w1351:string, "Index 0"=w1350:dbl, "Index 1"=w1349:dbl)  [unwired: 3 out]
          n460 = Not Equal To 0?(x=w1350) -> (x != 0?=w1358:bool)
          n461 = case shown="False" w1358 {
            tunnel: w1350 -> [_ w1362]
            tunnel: w1349 -> [_ w1361]
            tunnel: [0.0 w1360] -> w1357
            frame False {
            }
            frame True {
              n462 = Divide(x=w1362, y=w1361) -> (x/y=w1363:dbl)
              n463 = Multiply(x=w1363, y=1000.0) -> (x*y=w1360:dbl)
            }
          }
        }
        frame "GMU:Source:Meas Den Ratio" {
          n464 = call "Read_value_of_earlier_Ch.vi"("Desired Ch to Read"="GMU:Source:Meas Density", "Ch names"=w1371, "Present scan array"=w1372) -> ("Value"=w1367:dbl, "Scan comment"=w1366:string)  [unwired: 1 in]
          n465 = Equal?(x=w1367, y=w1365) -> (x = y?=w1369:bool)
          n466 = case shown="False" w1369 {
            tunnel: w1367 -> [w1374 _]
            tunnel: [w1373 w1379] -> w1368
            tunnel: w1365 -> [_ w1379]
            frame False {
              n467 = global read "Gas_management_global.vi" "Release temp (deg C)"() -> (w1377:dbl)
              n468 = global read "Gas_management_global.vi" "Atmos Pres (mbars)"() -> (w1376:dbl)
              n469 = call "Gas_Density.vi"("Pressure (mbar)"=w1376, "Temperature (C)"=w1377, "Gas"="Air" ("Gas Name")) -> ("Density (kg/m^3) (= g/l)"=w1375:dbl)
              n470 = Divide(x=w1374, y=w1375) -> (x/y=w1373:dbl)
            }
            frame True {
            }
          }
        }
        frame "GMU:Source:ppm/%Density" {
          # "Source ppm"
          # "% Delta Density of source"
          n471 = call "Read_value_of_earlier_Ch.vi"("Desired Ch to Read"="GMU:Source:Meas Strength", "Ch names"=w1393, "Present scan array"=w1394) -> ("Value"=w1391:dbl, "Scan comment"=w1395:string)  [unwired: 1 in]
          n472 = call "Read_value_of_earlier_Ch.vi"("Desired Ch to Read"="GMU:Source:Meas Den Ratio", "Ch names"=w1393, "Present scan array"=w1394) -> ("Value"=w1389:dbl)  [unwired: 1 in, 1 out]
          n473 = Subtract(x=w1389, y=1.0) -> (x-y=w1386:dbl)
          n474 = Multiply(x=w1391, y=10000.0) -> (x*y=w1387:dbl)
          n475 = Multiply(x=w1386, y=100.0) -> (x*y=w1380:dbl)
          n476 = Absolute Value(x=w1380) -> (abs(x)=w1381:dbl)
          n477 = Greater?(x=w1381, y=1.5) -> (0:w1383:bool)
          n478 = case shown="False" w1383 {
            tunnel: w1387 -> [_ w1400]
            tunnel: w1380 -> [_ w1399]
            tunnel: [nan w1398] -> w1382
            frame False {
            }
            frame True {
              n479 = Divide(x=w1400, y=w1399) -> (x/y=w1398:dbl)
            }
          }
        }
        frame "GMU:Source:Meas Strength" {
          n480 = call "Calculate_Release_Flowrates.vi"("Ch names"=w1416, "Units"=enum16{"Q l/min", "M_dot Kg/min"}."Q l/min", "Present scan array"=w1415) -> ("Trace"=w1408:dbl, "Carrier"=w1409:dbl, "Scan comments"=w1414:string)
          n481 = Equal To 0?(x=w1409) -> (x = 0?=w1411:bool)
          n482 = Equal To 0?(x=w1408) -> (x = 0?=w1412:bool)
          n483 = And(x=w1411, y=w1412) -> (x .and. y?=w1410:bool)
          n484 = case shown="False" w1410 {
            tunnel: w1409 -> [w1427 _]
            tunnel: w1408 -> [w1426 _]
            tunnel: [w1425 0.0] -> w1404
            frame False {
              n485 = Add(x=w1427, y=w1426) -> (x+y=w1430:dbl)
              n486 = Divide(x=w1426, y=w1430) -> (x/y=w1429:dbl)
              n487 = Multiply(x=w1429, y=100.0) -> (x*y=w1425:dbl)
            }
            frame True {
            }
          }
          n488 = while {
            tunnel: [w1418] -> w1401
            tunnel: [w1419] -> w1403
            tunnel: w1404 -> [w1424]
            shift-left: _ -> [w1418]
            shift-left: _ -> [w1423]
            shift-right: [w1424] -> _
            stop <- FALSE continue-if-true
            w1422 = 6.0 ("y")
            n489 = Less?(x=w1423, y=w1422) -> (x < y?=w1421:bool)
            n490 = Less?(x=w1418, y=w1422) -> (x < y?=w1420:bool)
            n491 = Or(x=w1421, y=w1420) -> (x .or. y?=w1419:bool)
          }
          n492 = Greater?(x=w1404, y=7.0) -> (0:w1402:bool)
          n493 = And(x=w1403, y=w1402) -> (x .and. y?=w1406:bool)
          n494 = Select(t=w1401, s=w1406, f=w1404) -> (s? t:f=w1405:dbl)
        }
        frame "EnFlo_Tunnel:Inlet_Temp:St Deviation" {
          n495 = global read "ADAM_Global.vi" "Active Ch names"() -> (w1442:string[])
          n496 = Unbundle By Name(w1438) -> ("A"=w1439:dbl)
          n497 = Less?(x=w1439, y=2.0) -> (x < y?=w1440:bool)
          n498 = case shown="True" w1440 {
            tunnel: w1436 -> [_ w1478]
            tunnel: w1437 -> [_ w1477]
            tunnel: string[] ["EnFlo_Tunnel:Inlet_Y=-1500:Z=50", "EnFlo_Tunnel:Inlet_Y=-1000:Z=50", "EnFlo_Tunnel:Inlet_Y=-500:Z=50", "EnFlo_Tunnel:Temp:Inlet_15_Bottom", "EnFlo_Tunnel:Inlet_Y=500:Z=50", "EnFlo_Tunnel:Inlet_Y=1000:Z=50", "EnFlo_Tunnel:Inlet_Y=1500:Z=50", "EnFlo_Tunnel:Inlet_Y=-1500:Z=450", "EnFlo_Tunnel:Inlet_Y=-1000:Z=450", "EnFlo_Tunnel:Inlet_Y=-500:Z=450", "EnFlo_Tunnel:Temp:Inlet_11", "EnFlo_Tunnel:Inlet_Y=500:Z=450", "EnFlo_Tunnel:Inlet_Y=1000:Z=450", "EnFlo_Tunnel:Inlet_Y=1500:Z=450", "EnFlo_Tunnel:Inlet_Y=-1500:Z=950", "EnFlo_Tunnel:Inlet_Y=-1000:Z=950", "EnFlo_Tunnel:Inlet_Y=-500:Z=950", "EnFlo_Tunnel:Temp:Inlet_6", "EnFlo_Tunnel:Inlet_Y=500:Z=950", "EnFlo_Tunnel:Inlet_Y=1000:Z=950", "EnFlo_Tunnel:Inlet_Y=1500:Z=950", "EnFlo_Tunnel:Inlet_Y=-1500:Z=1450", "EnFlo_Tunnel:Inlet_Y=-1000:Z=1450", "EnFlo_Tunnel:Inlet_Y=-500:Z=1450", "EnFlo_Tunnel:Temp:Inlet_1_Top", "EnFlo_Tunnel:Inlet_Y=500:Z=1450", "EnFlo_Tunnel:Inlet_Y=1000:Z=1450", "EnFlo_Tunnel:Inlet_Y=1500:Z=1450", "EnFlo_Tunnel:Setpoint:Inlet_15_Bottom", "EnFlo_Tunnel:Setpoint:Inlet_11", "EnFlo_Tunnel:Setpoint:Inlet_6", "EnFlo_Tunnel:Setpoint:Inlet_1_Top"] ("subarray") -> [w1447 w1476]
            tunnel: [w1445 w1474] -> w1434
            tunnel: w1442 -> [_ w1473]
            tunnel: [w1448 w1470] -> w1432
            tunnel: w1439 -> [w1449 _]
            frame False {
              w1455 = FALSE  # All Active Channels
              n499 = Get Date/Time In Seconds() -> (seconds since 1Jan1904=w1458:timestamp)
              n500 = To Double Precision Float(number=w1458) -> (double precision float=w1456:dbl)
              n501 = Subtract(x=w1456, y=w1449) -> (x-y=w1457:dbl)
              n502 = call "Get_ADAM_averages_server.vi"("No of averages"=1, "All Active Channels"=w1455, "End time"=w1456, "Start time"=w1457, "Clients time"=w1456, "ADAM Ch Names"=w1447) -> ("DBL values"=w1453:dbl[][])  [unwired: 4 out]
              n503 = Index Array(array=w1453, index (row)=0) -> (element=w1450:dbl[])  [unwired: 1 in]
              n504 = Array Subset(array=w1450, index=1) -> (w1444:dbl[])  [unwired: 1 in]
              n505 = call "Normalise Inlet Temps array.vi"("Temps plus setpoints"=w1444) -> ("Normalised Temps"=w1443:dbl[])
              n506 = for {
                tunnel: w1443 -> [w1464] mode=indexing
                tunnel: [w1464] -> w1448 mode=indexing if=w1462
                tunnel: w1447 -> [w1461] mode=indexing
                shift-right: [w1459] -> w1445
                shift-left: "" -> [w1460]
                n507 = Not A Number/Path/Refnum?(number/path/refnum=w1464) -> (NaN/Path/Refnum?=w1463:bool)
                n508 = Not(x=w1463) -> (.not. x?=w1462:bool)
                n509 = case shown="False" w1462 {
                  tunnel: w1461 -> [w1467 _]
                  tunnel: w1460 -> [w1466 w1469]
                  tunnel: [w1465 w1469] -> w1459
                  frame False {
                    n510 = Format Into String(format string="Channel \"%s\" is not currently active.\n", initial string=w1466, w1467) -> (resulting string=w1465:string)  [unwired: 1 in, 1 out]
                  }
                  frame True {
                  }
                }
              }
            }
            frame True {
              n511 = for {
                tunnel: w1478 -> [w1492]
                tunnel: w1477 -> [w1491]
                tunnel: w1476 -> [w1488] mode=indexing
                shift-right: [w1489] -> w1474
                shift-left: "" -> [w1490]
                tunnel: w1473 -> [w1483]
                tunnel: [w1482] -> w1472 mode=indexing
                n512 = call "Read_value_of_earlier_Ch.vi"("Desired Ch to Read"=w1488, "Ch names"=w1492, "Present scan array"=w1491) -> ("Value"=w1486:dbl, "Scan comment"=w1485:string)  [unwired: 1 in]
                n513 = Not A Number/Path/Refnum?(number/path/refnum=w1486) -> (NaN/Path/Refnum?=w1487:bool)
                n514 = case shown="False" w1487 {
                  tunnel: w1488 -> [w1495 _]
                  tunnel: [w1498 w1508] -> w1482
                  tunnel: w1486 -> [w1497 w1508]
                  tunnel: [w1500 w1507] -> w1484
                  tunnel: w1485 -> [w1499 w1507]
                  tunnel: w1483 -> [w1496 _]
                  frame False {
                    n515 = Search 1D Array(1D array=w1496, element=w1495) -> (index of element=w1493:i32)  [unwired: 1 in]
                    n516 = Greater Or Equal To 0?(x=w1493) -> (x >= 0?=w1494:bool)
                    n517 = case shown="False" w1494 {
                      tunnel: w1495 -> [w1504 _]
                      tunnel: [w1503 w1506] -> w1500
                      tunnel: w1499 -> [_ w1506]
                      tunnel: [nan w1505] -> w1498
                      tunnel: w1497 -> [_ w1505]
                      frame False {
                        n518 = Format Into String(format string="Channel \"%s\" is not currently active.\n", w1504) -> (resulting string=w1503:string)  [unwired: 2 in, 1 out]
                      }
                      frame True {
                      }
                    }
                  }
                  frame True {
                  }
                }
                n519 = Concatenate Strings(w1490, w1484) -> (w1489:string)
              }
              n520 = call "Normalise Inlet Temps array.vi"("Temps plus setpoints"=w1472) -> ("Normalised Temps"=w1471:dbl[])
              n521 = for {
                tunnel: w1471 -> [w1480] mode=indexing
                tunnel: [w1480] -> w1470 mode=indexing if=w1479
                n522 = Not A Number/Path/Refnum?(number/path/refnum=w1480) -> (NaN/Path/Refnum?=w1481:bool)
                n523 = Not(x=w1481) -> (.not. x?=w1479:bool)
              }
            }
          }
          n524 = call <vilib>:"Std Deviation and Variance.vi"("X"=w1432) -> ("standard deviation"=w1433:dbl)  [unwired: 1 in, 2 out]
        }
        frame "EnFlo Lab:labstrat1:Delta T" {
          n525 = Build Array("EnFlo Lab:labstrat1:Z=4.5m", "EnFlo Lab:labstrat1:Z=0.5m") -> (w1516:string[])
          n526 = call "Read_Earlier_Channels.vi"("Present scan array"=w1512, "Ch names"=w1513, "Desired Channels"=w1516) -> ("Scan comments"=w1511:string, "Index 0"=w1510:dbl, "Index 1"=w1509:dbl)  [unwired: 3 out]
          n527 = Subtract(x=w1510, y=w1509) -> (x-y=w1517:dbl)
        }
        frame "EnFlo_Tunnel:Chilled Water:Valve Dem Pos" {
          n528 = while {
            shift-right: [w1531] -> _
            shift-left: _ -> [w1533]
            tunnel: w1523 -> [w1532]
            tunnel: w1522 -> [w1530]
            tunnel: w1521 -> [w1529]
            tunnel: w1520 -> [w1528]
            tunnel: [w1527] -> w1519
            tunnel: [w1526] -> w1518
            shift-right: [w1525] -> _
            shift-left: _ -> [w1524]
            stop <- TRUE stop-if-true
            # "Av Pos"
            # "Need\nCool"
            # "Current"
            # "Dem"
            # "Run PID"
            n529 = stacked-sequence {
              seq-local: [w1544 _ _] -> [_ _ w1586]
              seq-local: [_ w1570 _] -> [_ _ w1583]
              seq-local: [_ w1569 _] -> [_ _ w1580]
              seq-local: [_ w1568 _] -> [_ _ w1579]
              seq-local: [w1535 _ _] -> [_ _ w1577]
              seq-local: [_ w1552 _] -> [_ _ w1576]
              tunnel: w1533 -> [w1542 _ _]
              tunnel: w1532 -> [w1549 _ _]
              tunnel: [w1541 _ _] -> w1531
              tunnel: w1530 -> [_ w1575 w1585]
              tunnel: w1529 -> [_ w1574 w1584]
              tunnel: w1528 -> [w1537 _ w1582]
              tunnel: [_ _ w1581] -> w1527
              tunnel: [_ _ w1578] -> w1526
              tunnel: [w1539 _ _] -> w1525
              tunnel: w1524 -> [w1538 _ _]
              frame #0 {
                n530 = Get Date/Time In Seconds() -> (seconds since 1Jan1904=w1550:timestamp)
                n531 = Unbundle By Name(w1549) -> ("A"=w1548:dbl)
                n532 = To Double Precision Float(number=w1550) -> (double precision float=w1543:dbl)
                n533 = Build Array (concatenate)(w1538, w1537) -> (w1536:dbl[])
                n534 = Subtract(x=w1543, y=w1542) -> (x-y=w1547:dbl)
                n535 = Greater?(x=w1547, y=w1548) -> (0:w1546:bool)
                n536 = Not A Number/Path/Refnum?(number/path/refnum=w1547) -> (NaN/Path/Refnum?=w1545:bool)
                n537 = call-poly <vilib>:"Mean.vi"("X"=w1536) -> ("mean"=w1535:dbl)  [unwired: 1 out]
                n538 = Or(x=w1545, y=w1546) -> (x .or. y?=w1544:bool)
                n539 = Select(t=w1543, s=w1544, f=w1542) -> (s? t:f=w1541:dbl)
                n540 = Array Subset(array=w1536, length="History Length") -> (w1539:dbl[])  [unwired: 1 in]
              }
              frame #1 {
                n541 = Build Array("EnFlo_Tunnel:Chilled Water:Dem Temp", "EnFlo_Tunnel:Chilled Water:Supply", "EnFlo_Tunnel:Floor_Cooling:Enable", "EnFlo_Tunnel:Heat_Ex_Div_Valve:Dem Pos") -> (w1571:string[])
                n542 = call "Read_Earlier_Channels.vi"("Present scan array"=w1575, "Ch names"=w1574, "Desired Channels"=w1571) -> ("Scan comments"=w1568:string, "Index 0"=w1570:dbl, "Index 1"=w1569:dbl, "Index 2"=w1562:dbl, "Index 3"=w1561:dbl)  [unwired: 1 out]
                n543 = Greater Than 0?(x=w1561) -> (x > 0?=w1565:bool)
                n544 = Greater?(x=w1562, y=0.5) -> (0:w1564:bool)
                n545 = Or(x=w1564, y=w1565) -> (x .or. y?=w1558:bool)
                n546 = Select(t=1.0, s=w1558, f=0.0) -> (s? t:f=w1555:dbl)
                n547 = feedback #1() -> (w1559:dbl[])  [unwired: 1 in]
                n548 = call "Running_Ch_Average.vi"("Shift In"=w1559, "History length"=600, "New Value"=w1555) -> ("Shift Out"=w1560:dbl[], "mean"=w1554:dbl)  [unwired: 3 in]
                n549 = feedback-in #1(w1560) -> ()
                n550 = Greater?(x=w1554, y=0.001) -> (0:w1552:bool)
              }
              frame #2 {
                n551 = case shown="True" w1586 {
                  tunnel: w1585 -> [_ w1608]
                  tunnel: w1584 -> [_ w1607]
                  tunnel: w1583 -> [_ w1605]
                  tunnel: w1582 -> [w1588 w1604]
                  tunnel: [w1588 w1600] -> w1581
                  tunnel: w1580 -> [_ w1599]
                  tunnel: w1579 -> [w1587 w1598]
                  tunnel: [w1587 w1596] -> w1578
                  tunnel: w1577 -> [_ w1591]
                  tunnel: w1576 -> [_ w1590]
                  frame False {
                  }
                  frame True {
                    n552 = call "Read_Earlier_Channels.vi"("Present scan array"=w1608, "Ch names"=w1607, "Desired Channels"=string[] ["EnFlo_Tunnel:Chiller_Pump:Running", "EnFlo_Tunnel:Chiller_Pump:Enable", "Uni:Chilled Water:Temp", "EnFlo_Tunnel:Chilled Water:Return"] ("appended array")) -> ("Scan comments"=w1597:string, "Index 0"=w1593:dbl, "Index 1"=w1601:dbl, "Index 2"=w1592:dbl, "Index 3"=w1589:dbl)  [unwired: 1 out]
                    n553 = Greater?(x=w1601, y=0.5) -> (0:w1602:bool)
                    n554 = Greater?(x=w1593, y=0.5) -> (0:w1594:bool)
                    n555 = case shown="True" w1594 {
                      tunnel: [w1621 w1631] -> w1600
                      tunnel: w1605 -> [_ w1629]
                      tunnel: w1599 -> [_ w1632]
                      tunnel: w1602 -> [w1620 _]
                      tunnel: w1604 -> [_ w1628]
                      tunnel: w1592 -> [_ w1630]
                      tunnel: w1591 -> [_ w1627]
                      tunnel: w1590 -> [_ w1626]
                      tunnel: w1589 -> [_ w1625]
                      frame False {
                        n556 = Seconds To Date/Time() -> (date time rec=w1609:T14)  [unwired: 2 out]
                        n557 = Unbundle By Name(w1609) -> ("day of week"=w1615:i32, "hour"=w1617:i32)
                        n558 = Less?(x=w1617, y=3) -> (x < y?=w1612:bool)
                        n559 = Equal?(x=7, y=w1615) -> (x = y?=w1613:bool)
                        n560 = And(x=w1613, y=w1612) -> (x .and. y?=w1611:bool)
                        n561 = case shown="False" w1620 {
                          tunnel: w1611 -> [w1622 w1624]
                          tunnel: [w1622 w1623] -> w1610
                          frame False {
                          }
                          frame True {
                            n562 = Not(x=w1624) -> (.not. x?=w1623:bool)
                          }
                        }
                        n563 = Select(t=0.0, s=w1610, f=100.0) -> (s? t:f=w1621:dbl)
                      }
                      frame True {
                        n564 = case shown="True" w1626 {
                          tunnel: w1632 -> [_ w1652]
                          tunnel: [0.0 ("Max") w1651] -> w1631
                          tunnel: w1630 -> [_ w1645]
                          tunnel: w1629 -> [_ w1640]
                          tunnel: w1628 -> [_ w1644]
                          tunnel: w1627 -> [_ w1642]
                          tunnel: w1625 -> [_ w1641]
                          frame False {
                          }
                          frame True {
                            w1653 = 100.0  # Max
                            w1654 = 0.0  # Min
                            n565 = call "PID.vi"("Present Value"=w1652, "Previous Scan Value"=w1644, "Setpoint"=w1640) -> ("Dem Output"=w1650:dbl)
                            n566 = Divide(x=w1642, y=100.0) -> (x/y=w1636:dbl)
                            n567 = Subtract(x=w1645, y=8.5) -> (x-y=w1646:dbl)
                            n568 = Subtract(x=1.0, y=w1636) -> (x-y=w1635:dbl)
                            n569 = Compound Arithmetic op=MULTIPLY(w1646, w1636, "K_Uni_chilled water") -> (w1647:dbl)
                            n570 = Subtract(x=w1641, y=w1640) -> (x-y=w1639:dbl)
                            n571 = Compound Arithmetic op=MULTIPLY(w1639, w1635, "K_Uni_chilled water") -> (w1634:dbl)
                            n572 = Compound Arithmetic op=ADD(w1634, w1650, w1647) -> (w1649:dbl)
                            n573 = In Range and Coerce(upper limit=w1653, x=w1649, lower limit=w1654) -> (coerced(x)=w1651:dbl)  [unwired: 1 out]
                          }
                        }
                      }
                    }
                    n574 = Concatenate Strings(w1597, w1598) -> (w1596:string)
                  }
                }
              }
            }
          }
        }
        frame "EnFlo_Tunnel:Hydrosonic:Integral" {
          n575 = Build Array("EnFlo_Tunnel:Reference:Velocity", "Hydrosonic:Transducer:Setting") -> (w1664:string[])
          n576 = call "Read_Earlier_Channels.vi"("Present scan array"=w1665, "Ch names"=w1663, "Desired Channels"=w1664) -> ("Scan comments"=w1657:string, "Index 0"=w1662:dbl, "Index 1"=w1656:dbl)  [unwired: 3 out]
          n577 = Greater?(x=w1662, y=0.5) -> (0:w1660:bool)
          n578 = case shown="True" w1660 {
            tunnel: w1659 -> [w1668 w1676]
            tunnel: [w1668 w1675] -> w1658
            tunnel: w1656 -> [_ w1674]
            tunnel: w1655 -> [_ w1673]
            frame False {
            }
            frame True {
              w1671 = 8640000.0  # Seconds per day x 100
              n579 = Multiply(x=w1674, y=w1673) -> (x*y=w1672:dbl)
              n580 = Divide(x=w1672, y=w1671) -> (x/y=w1670:dbl)
              n581 = Not A Number/Path/Refnum?(number/path/refnum=w1670) -> (NaN/Path/Refnum?=w1669:bool)
              n582 = case shown="False" w1669 {
                tunnel: w1676 -> [w1679 w1680]
                tunnel: [w1678 w1680] -> w1675
                tunnel: w1670 -> [w1677 _]
                frame False {
                  n583 = Add(x=w1677, y=w1679) -> (x+y=w1678:dbl)
                }
                frame True {
                }
              }
            }
          }
        }
        frame "EnFlo_Tunnel:Ref Pitot:Velocity" {
          # "Temp"
          n584 = stacked-sequence {
            seq-local: [w1692 _] -> [_ w1720]
            seq-local: [w1685 _] -> [_ w1718]
            tunnel: w1684 -> [w1700 w1714]
            tunnel: w1683 -> [w1699 w1715]
            tunnel: [_ w1719] -> w1682
            tunnel: [_ w1716] -> w1681
            frame #0 {
              w1702 = 50.0 ("y")
              w1703 = 100.0 ("y")
              n585 = call "Read_value_of_earlier_Ch.vi"("Desired Ch to Read"="EnFlo_Tunnel:Ref Pitot:Z (mm)", "Ch names"=w1699, "Present scan array"=w1700) -> ("Value"=w1695:dbl, "Scan comment"=w1687:string)  [unwired: 1 in]
              n586 = Divide(x=w1695, y=w1703) -> (x/y=w1704:dbl)
              n587 = Round To Nearest(number=w1704) -> (nearest integer value=w1691:dbl)
              n588 = In Range and Coerce(upper limit=13.0, x=w1691, lower limit=1.0) -> (coerced(x)=w1688:dbl)  [unwired: 1 out]
              n589 = Multiply(x=w1688, y=w1703) -> (x*y=w1701:dbl)
              n590 = Subtract(x=w1701, y=w1702) -> (x-y=w1698:dbl)
              n591 = Add(x=w1701, y=w1702) -> (x+y=w1697:dbl)
              n592 = Build Array(w1698, w1697) -> (w1696:dbl[])
              n593 = for {
                tunnel: w1700 -> [w1713]
                tunnel: w1699 -> [w1711]
                tunnel: w1696 -> [w1709] mode=indexing
                tunnel: [w1707] -> w1693 mode=indexing
                tunnel: [w1706] -> w1686 mode=indexing
                n594 = Number To Decimal String(number=w1709) -> (decimal integer string=w1708:string)  [unwired: 1 in]
                n595 = Concatenate Strings("EnFlo_Tunnel:Temp:Inlet_Y=0_Z=", w1708) -> (w1712:string)
                n596 = call "Read_value_of_earlier_Ch.vi"("Desired Ch to Read"=w1712, "Ch names"=w1711, "Present scan array"=w1713) -> ("Value"=w1707:dbl, "Scan comment"=w1706:string)  [unwired: 1 in]
              }
              n597 = Threshold 1D Array(2:w1695, 3:w1696) -> (0:w1694:dbl)  [unwired: 1 in]
              n598 = Interpolate 1D Array(1:w1694, 2:w1693) -> (0:w1692:dbl)
              n599 = Concatenate Strings(w1687, w1686) -> (w1685:string)
            }
            frame #1 {
              n600 = Build Array("EnFlo_Tunnel:Ref Pitot Pdyn SDP610:(Pa)", "EnFlo_Tunnel:Ref Pitot Zero SDP610:(Pa)", "Froude:NPL:Atmos_Press", "EnFlo_Tunnel:Ref Pitot Zero:Enable") -> (w1733:string[])
              n601 = call "Read_Earlier_Channels.vi"("Present scan array"=w1714, "Ch names"=w1715, "Desired Channels"=w1733) -> ("Scan comments"=w1717:string, "Index 0"=w1724:dbl, "Index 1"=w1723:dbl, "Index 2"=w1721:dbl, "Index 3"=w1727:dbl)  [unwired: 1 out]
              n602 = Greater?(x=w1727, y=0.5) -> (0:w1726:bool)
              n603 = while {
                shift-right: [w1751] -> _
                shift-left: _ -> [w1750]
                shift-left: _ -> [w1749]
                shift-left: _ -> [w1748]
                shift-left: _ -> [w1747]
                tunnel: w1726 -> [w1751]
                tunnel: [w1745] -> w1725
                stop <- TRUE stop-if-true
                n604 = Compound Arithmetic op=OR(w1751, w1750, w1749, w1748, w1747) -> (invert w1745:bool)
              }
              n605 = Subtract(x=w1724, y=w1723) -> (x-y=w1722:dbl)
              n606 = case shown="True" w1725 {
                tunnel: w1722 -> [_ w1739]
                tunnel: w1721 -> [_ w1741]
                tunnel: w1720 -> [_ w1740]
                tunnel: [nan w1737] -> w1719
                frame False {
                }
                frame True {
                  n607 = Absolute Value(x=w1739) -> (abs(x)=w1735:dbl)
                  n608 = formula code="Rho=(Patmos*100)/(287*(T+273));\nU=sqrt(2*Pdyn/Rho);"("Patmos"=w1741, "T"=w1740, "Pdyn"=w1735) -> ("U"=w1736:dbl)  [unwired: 1 out]
                  n609 = Greater Than 0?(x=w1739) -> (x > 0?=w1738:bool)
                  n610 = case shown="True" w1738 {
                    tunnel: [w1742 w1744] -> w1737
                    tunnel: w1736 -> [w1743 w1744]
                    frame False {
                      n611 = Negate(x=w1743) -> (-x=w1742:dbl)
                    }
                    frame True {
                    }
                  }
                }
              }
              n612 = Concatenate Strings(w1717, w1718) -> (w1716:string)
            }
          }
        }
        frame "EnFlo_Tunnel:Days Run at:2.5m/s" {
          n613 = Build Array("EnFlo_Tunnel:Reference:Velocity") -> (w1760:string[])
          n614 = call "Read_Earlier_Channels.vi"("Present scan array"=w1761, "Ch names"=w1759, "Desired Channels"=w1760) -> ("Scan comments"=w1754:string, "Index 0"=w1752:dbl)  [unwired: 4 out]
          n615 = Greater?(x=w1752, y=0.5) -> (0:w1757:bool)
          n616 = case shown="True" w1757 {
            tunnel: w1756 -> [w1763 w1771]
            tunnel: [w1763 w1770] -> w1755
            tunnel: w1752 -> [_ w1769]
            tunnel: w1753 -> [_ w1768]
            frame False {
            }
            frame True {
              w1766 = 216000.0  # Seconds per day x 2.5
              n617 = Multiply(x=w1769, y=w1768) -> (x*y=w1767:dbl)
              n618 = Divide(x=w1767, y=w1766) -> (x/y=w1765:dbl)
              n619 = Not A Number/Path/Refnum?(number/path/refnum=w1765) -> (NaN/Path/Refnum?=w1764:bool)
              n620 = case shown="True" w1764 {
                tunnel: w1771 -> [w1774 w1775]
                tunnel: [w1773 w1775] -> w1770
                tunnel: w1765 -> [w1772 _]
                frame False {
                  n621 = Add(x=w1772, y=w1774) -> (x+y=w1773:dbl)
                }
                frame True {
                }
              }
            }
          }
        }
        frame "Complete:Scan:Period" {
          n622 = while {
            tunnel: [w1785] -> w1778
            tunnel: [w1792] -> w1780
            shift-left: _ -> [w1792]
            shift-right: [w1793] -> w1781
            tunnel: w1777 -> [w1789]
            tunnel: [w1784] -> w1776
            stop <- FALSE continue-if-true
            w1784 = 10.0 ("Averaging time (mins)")
            n623 = Build Array(w1789) -> (w1788:string[])
            n624 = call "Get_Channel_averages.vi"("Desired Ch Names"=w1788, "Averaging time (mins)"=w1784) -> ("number"=w1787:dbl[])  [unwired: 1 in, 2 out]
            n625 = Index Array(array=w1787, index=0) -> (element=w1785:dbl)
            n626 = Greater?(x=w1785, y=20.0) -> (0:w1793:bool)
          }
          n627 = Compound Arithmetic op=AND(w1781, invert w1780) -> (w1779:bool)
          n628 = case shown="True" w1779 {
            tunnel: w1778 -> [_ w1799]
            tunnel: w1776 -> [_ w1794]
            frame False {
            }
            frame True {
              n629 = Format Into String(format string="Warning! The average scan period on the ADAM Scan table is %.1f seconds over the last %d minutes." ("Format String"), w1799, w1794) -> (resulting string=w1797:string)  [unwired: 2 in, 1 out]
              n630 = call "Server_Emails.vi"("Message"=w1797, "Contact All clients?"=TRUE, "Subject"="Scan Period") -> ()  [unwired: 2 in, 3 out]
            }
          }
        }
        frame "GMU:Source:Est Time" {
          # "NaN's"
          # "Est?"
          # "Inband?"
          n631 = stacked-sequence {
            seq-local: [w1806 _ _ _] -> [_ _ w1853 _]
            seq-local: [_ w1818 _ _] -> [_ _ w1850 _]
            seq-local: [_ w1819 _ _] -> [_ _ w1848 _]
            seq-local: [_ _ w1855 _] -> [_ _ _ w1871]
            seq-local: [w1810 _ _ _] -> [_ _ w1852 _]
            seq-local: [_ w1817 _ _] -> [_ _ _ w1867]
            tunnel: w1805 -> [w1812 w1820 w1858 _]
            tunnel: w1804 -> [w1811 w1821 w1859 _]
            tunnel: [_ _ w1851 _] -> w1803
            tunnel: [_ _ _ w1870] -> w1802
            tunnel: w1801 -> [_ _ _ w1869]
            tunnel: w1800 -> [_ _ _ w1868]
            frame #0 {
              n632 = Build Array("GMU:Carrier 1:Dem Q", "GMU:Carrier 2:Dem Q", "GMU:Trace:Dem Q") -> (w1813:string[])
              n633 = call "Read_Earlier_Channels.vi"("Present scan array"=w1811, "Ch names"=w1812, "Desired Channels"=w1813) -> ("Scan comments"=w1810:string, "Index 0"=w1809:dbl, "Index 1"=w1808:dbl, "Index 2"=w1807:dbl)  [unwired: 2 out]
              n634 = Build Array(w1809, w1808, w1807) -> (w1806:dbl[])
            }
            frame #1 {
              n635 = for {
                N: 2 -> [_]
                tunnel: w1821 -> [w1831]
                tunnel: w1820 -> [w1832]
                tunnel: [w1830] -> w1818 mode=indexing
                tunnel: [w1837] -> w1819 mode=indexing
                tunnel: [w1836] -> w1817 mode=indexing
                i -> [w1842]
                w1841 = 23.0  # %
                n636 = case shown="0, Default" w1842 {
                  tunnel: ["GMU:Source:Meas Q" "GMU:Source:Meas Strength"] -> w1835
                  tunnel: ["GMU:Source:Dem Q" "GMU:Source:Dem Strength"] -> w1834
                  frame 0, Default {
                  }
                  frame 1 {
                  }
                }
                n637 = Build Array(w1834, w1835) -> (w1833:string[])
                n638 = call "Read_Earlier_Channels.vi"("Present scan array"=w1831, "Ch names"=w1832, "Desired Channels"=w1833) -> ("Scan comments"=w1830:string, "Index 0"=w1828:dbl, "Index 1"=w1829:dbl)  [unwired: 3 out]
                n639 = Not A Number/Path/Refnum?(number/path/refnum=w1829) -> (NaN/Path/Refnum?=w1836:bool)
                n640 = Subtract(x=w1829, y=w1828) -> (x-y=w1827:dbl)
                n641 = Greater Than 0?(x=w1828) -> (x > 0?=w1838:bool)
                n642 = Less?(x=w1827, y=0.05) -> (x < y?=w1824:bool)
                n643 = call "In_Range_check.vi"("%"=w1841, "Mode"=In_Range."%", "Value"=w1829, "Setpoint"=w1828) -> ("In Range"=w1825:bool)  [unwired: 1 in, 2 out]
                n644 = Or(x=w1825, y=w1824) -> (x .or. y?=w1823:bool)
                n645 = And(x=w1823, y=w1838) -> (x .and. y?=w1839:bool)
                n646 = Compound Arithmetic op=OR(w1839, invert w1838, w1836) -> (w1837:bool)
              }
            }
            frame #2 {
              n647 = while {
                tunnel: [w1866] -> w1854
                tunnel: w1853 -> [w1865]
                shift-left: _ -> [w1866]
                shift-right: [w1865] -> _
                stop <- FALSE continue-if-true
              }
              n648 = Equal?(x=w1853, y=w1854) -> (x = y?=w1860:bool)
              n649 = call "Read_value_of_earlier_Ch.vi"("Desired Ch to Read"="GMU:Source:Dem Q", "Ch names"=w1858, "Present scan array"=w1859) -> ("Value"=w1856:dbl)  [unwired: 1 in, 1 out]
              n650 = Greater Than 0?(x=w1856) -> (x > 0?=w1863:bool)
              n651 = And Array Elements(Boolean array=w1848) -> (logical AND=w1847:bool)
              n652 = Select(t=w1847, s=w1863, f=TRUE) -> (s? t:f=w1861:bool)
              n653 = Compound Arithmetic op=AND(w1860, w1861) -> (w1855:bool)
              n654 = Concatenate Strings(w1850) -> (w1849:string)
              n655 = Concatenate Strings(w1849, w1852) -> (w1851:string)
            }
            frame #3 {
              n656 = case shown="False" w1871 {
                tunnel: [0.0 w1873] -> w1870
                tunnel: w1869 -> [_ w1878]
                tunnel: w1868 -> [_ w1874]
                tunnel: w1867 -> [_ w1877]
                frame False {
                }
                frame True {
                  n657 = Or Array Elements(Boolean array=w1877) -> (logical OR=w1876:bool)
                  n658 = Add(x=w1878, y=w1874) -> (x+y=w1875:dbl)
                  n659 = Select(t=w1874, s=w1876, f=w1875) -> (s? t:f=w1873:dbl)
                }
              }
            }
          }
        }
      }
    }
    frame "AutoZero" {
      n660 = call "CPP-ZeroMonitor.vi"("Scan Period"=w1883, "Previous Scan Value"=w1879, "Present scan array"=w1884, "Value to Output"=w1882, "Ch Description"=w1885, "Ch names"=w1886) -> ("Scan comment"=w1881:string, "Output"=w1880:dbl)  [unwired: 1 in, 1 out]
    }
    frame "Average", "St Deviation" {
      n661 = call "Stats.vi"("Scan Period"=w1890, "Present scan array"=w1889, "Ch Description"=w1892, "Ch names"=w1891) -> ("String"=w1887:string, "Stat"=w1888:dbl)  [unwired: 3 in, 1 out]
    }
    frame "Coded" {
    }
    frame "Client Info" {
      n662 = global read "ADAM_Global.vi" "Client State Array"() -> (w1907:T15[])
      n663 = call "Split_Ch_name.vi"("Ch name"=w1901) -> ("Top level"=w1899:string, "Low level"=w1897:string)  [unwired: 1 out]
      n664 = Equal?(x="Status" ("Substring"), y=w1899) -> (x = y?=w1898:bool)
      n665 = Select(t=w1897, s=w1898, f="") -> (s? t:f=w1895:string)
      n666 = for {
        tunnel: w1907 -> [w1916] mode=indexing
        tunnel: [w1915] -> w1908 mode=indexing
        n667 = Unbundle By Name(w1916) -> ("Client Name"=w1915:string)
      }
      n668 = Search 1D Array(1D array=w1908, element=w1895) -> (index of element=w1903:i32)  [unwired: 1 out]
      n669 = Less Than 0?(x=w1903) -> (x < 0?=w1902:bool)
      n670 = Index Array(array=w1907, index=w1903) -> (element=w1906:T15)
      n671 = case shown="False" w1902 {
        tunnel: w1906 -> [w1911 _]
        tunnel: w1895 -> [w1910 w1913]
        tunnel: [w1909 w1912] -> w1905
        frame False {
          n672 = call "Get_Client_Status_string.vi"("Client State Cluster"=w1911, "Client Name"=w1910) -> ("Code Value"=w1909:dbl)  [unwired: 1 in]
        }
        frame True {
          w1912 = 7.0 ("Code Value")
          n673 = call "Remember_value.vi"("Mode"=Remember_value_mode."Read and Write", "Input Value"=w1912, "Ch name"=w1913) -> ()  [unwired: 1 out]
        }
      }
    }
    frame "Comparator" {
      n674 = call "Comparator.vi"("Previous Scan Value"=w1917, "Present scan array"=w1920, "Ch Description"=w1921, "Ch names"=w1922) -> ("String"=w1918:string, "Value"=w1919:dbl)  [unwired: 3 in, 1 out]
    }
    frame "Equation" {
      n675 = call "CPP-Equation.vi"("Scan Period"=w1927, "Previous Scan Value"=w1923, "Present scan array"=w1928, "Value to Output"=w1926, "Ch Description"=w1929, "Ch names"=w1930) -> ("Scan comment"=w1925:string, "Output"=w1924:dbl)  [unwired: 1 in, 1 out]
    }
    frame "Hold Value" {
    }
    frame "Read Ch" {
      n676 = Unbundle By Name(w1936) -> ("String"=w1933:string)
      n677 = call "Read_value_of_earlier_Ch.vi"("Desired Ch to Read"=w1933, "Ch names"=w1937, "Present scan array"=w1938) -> ("Value"=w1934:dbl, "Scan comment"=w1935:string)  [unwired: 1 in]
    }
    frame "Read A" {
      n678 = Unbundle By Name(w1940) -> ("A"=w1939:dbl)
    }
    frame "ScanPacer" {
      # "Computes delay to use to achieve \"A\" ms scan period"
      n679 = call "ADAMPacer.vi"("Scan Period"=w1942, "Previous Scan Value"=w1943, "Ch Description"=w1946) -> ("Scan comment"=w1944:string, "Output"=w1945:dbl)  [unwired: 4 in, 1 out]
    }
    frame "Count Down Timer" {
      n680 = Equal To 0?(x=w1948) -> (x = 0?=w1947:bool)
      n681 = case shown="False" w1947 {
        tunnel: w1951 -> [w1961 _]
        tunnel: [w1958 w1965] -> w1950
        tunnel: w1948 -> [w1959 w1965]
        frame False {
          n682 = Absolute Value(x=w1959) -> (abs(x)=w1960:dbl)
          n683 = Greater Than 0?(x=w1959) -> (x > 0?=w1954:bool)
          n684 = Subtract(x=w1960, y=w1961) -> (x-y=w1957:dbl)
          n685 = Less Than 0?(x=w1957) -> (x < 0?=w1952:bool)
          n686 = Select(t=0.0, s=w1952, f=w1957) -> (s? t:f=w1955:dbl)
          n687 = Or(x=w1952, y=w1954) -> (x .or. y?=w1953:bool)
          n688 = case shown="True" w1953 {
            tunnel: [w1962 w1964] -> w1958
            tunnel: w1955 -> [w1963 w1964]
            frame False {
              n689 = Negate(x=w1963) -> (-x=w1962:dbl)
            }
            frame True {
            }
          }
        }
        frame True {
        }
      }
    }
    frame "Test" {
      n690 = Get Date/Time In Seconds() -> (seconds since 1Jan1904=w1966:timestamp)
      n691 = To Double Precision Float(number=w1966) -> (double precision float=w1971:dbl)
      n692 = Subtract(x=w1971, y=2969882881.0) -> (x-y=w1970:dbl)
      n693 = Multiply(x=w1970, y=0.0005) -> (x*y=w1967:dbl)
      n694 = Random Number (0-1)() -> (number: 0 to 1=w1968:dbl)
      n695 = Add(x=w1968, y=w1967) -> (x+y=w1974:dbl)
    }
    frame "Web Client" {
      w1984 = 7200.0  # 2 Hours in Seconds
      n696 = Concatenate Strings(w1993, ":Last read" ("Substring")) -> (w1991:string)
      n697 = call "Remember_value.vi"("Mode"=Remember_value_mode."Read only", "Ch name"=w1991) -> ("Output Value"=w1990:dbl)  [unwired: 1 in]
      n698 = Not A Number/Path/Refnum?(number/path/refnum=w1990) -> (NaN/Path/Refnum?=w1988:bool)
      n699 = Get Date/Time In Seconds() -> (seconds since 1Jan1904=w1983:timestamp)
      n700 = To Double Precision Float(number=w1983) -> (double precision float=w1981:dbl)
      n701 = Subtract(x=w1981, y=w1990) -> (x-y=w1996:dbl)
      n702 = Greater?(x=w1996, y=1800.0) -> (0:w1989:bool)
      n703 = Or(x=w1989, y=w1988) -> (x .or. y?=w1975:bool)
      n704 = case shown="True" w1975 {
        frame False {
        }
        frame True {
          n705 = global read "Constants_global.vi" "EnFlo SW Folder"() -> (w1999:path)
          n706 = Build Path(base path=w1999, name or relative path=path "ADAM Server/SoftwareChannels/Web_Client.vi") -> (appended path=w1998:path)
          n707 = Open VI Reference(vi path=w1998) -> (vi reference=w2003:refnum<vi>, error out=w2004:errorcluster)  [unwired: 1 in, 4 out]
          n708 = property class="VI"(reference=w2003, error in=w2004) -> (reference out=w2006:refnum<vi>, error out=w2007:errorcluster, "Front Panel Window:Open"=w2005:bool)
          n709 = case shown="False" w2005 {
            tunnel: w2006 -> [w2013 w2016]
            tunnel: w2007 -> [w2012 w2015]
            tunnel: [w2011 w2016] -> w2008
            tunnel: [w2010 w2015] -> w2009
            frame False {
              n710 = property class="VI"(reference=w2013, error in=w2012, "Front Panel Window:Open"=TRUE) -> (reference out=w2011:refnum<vi>, error out=w2010:errorcluster)
            }
            frame True {
            }
          }
          n711 = invoke class="VI" method="Run VI"(reference=w2008, error in=w2009, "Wait until done"=FALSE, "Auto Dispose Ref"=TRUE) -> ()  [unwired: 1 in, 5 out]
        }
      }
      n712 = Concatenate Strings(w1993, ":value time" ("Substring")) -> (w1977:string)
      n713 = call "Remember_value.vi"("Mode"=Remember_value_mode."Read only", "Ch name"=w1993) -> ("Output Value"=w1997:dbl)  [unwired: 1 in]
      n714 = call "Remember_value.vi"("Mode"=Remember_value_mode."Read only", "Ch name"=w1977) -> ("Output Value"=w1982:dbl)  [unwired: 1 in]
      n715 = Subtract(x=w1981, y=w1982) -> (x-y=w1980:dbl)
      n716 = Greater?(x=w1980, y=w1984) -> (0:w1987:bool)
      n717 = case shown="True" w1987 {
        tunnel: w1980 -> [_ w2022]
        tunnel: 3600.0 ("y") -> [_ w2021]
        tunnel: ["" w2019] -> w1986
        frame False {
        }
        frame True {
          n718 = Divide(x=w2022, y=w2021) -> (x/y=w2018:dbl)
          n719 = Format Into String(format string="Value is %d hours old." ("Format String"), w2018) -> (resulting string=w2019:string)  [unwired: 2 in, 1 out]
        }
      }
    }
    frame "Run VI Named:" {
      n720 = Current VI's Path() -> (path=w2041:path)
      n721 = call <vilib>:"Trim Whitespace.vi"("string"=w2024) -> ("trimmed string"=w2023:string)  [unwired: 1 in]
      n722 = Strip Path(path=w2041) -> (stripped path=w2042:path)  [unwired: 1 out]
      n723 = Strip Path(path=w2042) -> (stripped path=w2043:path)  [unwired: 1 out]
      n724 = Build Path(base path=w2043, name or relative path="Run_vi_named") -> (appended path=w2045:path)
      n725 = Build Path(base path=w2045, name or relative path=w2023) -> (appended path=w2040:path)
      n726 = Open VI Reference(type specifier VI Refnum (for type only)=refnum<vi> refnum, vi path=w2040) -> (vi reference=w2036:refnum<vi>, error out=w2035:errorcluster)  [unwired: 1 in, 3 out]
      n727 = property class="VI Interface Type 0"(reference=w2036, error in=w2035) -> (reference out=w2038:refnum<vi>, error out=w2037:errorcluster, "Front Panel Window:Open"=w2039:bool)
      n728 = case shown="False" w2039 {
        tunnel: w2038 -> [w2053 w2055]
        tunnel: w2037 -> [w2052 w2054]
        tunnel: [w2051 w2055] -> w2034
        tunnel: [w2049 w2054] -> w2033
        frame False {
          n729 = property class="VI Interface Type 0"(reference=w2053, error in=w2052, "Front Panel Window:Open"=TRUE) -> (reference out=w2051:refnum<vi>, error out=w2049:errorcluster)
        }
        frame True {
        }
      }
      n730 = call-by-ref "?"(reference=w2034, error in=w2033, "Scan Period"=w2027, "Previous Scan Value"=w2028, "Present scan array"=w2029, "Value to Output"=w2030, "Ch Description"=w2031, "Ch names"=w2032) -> (reference out=w2047:refnum<vi>, error out=w2048:errorcluster, "Scan comment"=w2025:string, "Output"=w2026:dbl)  [unwired: 2 in]
      n731 = Close Reference(reference=w2047, error in (no error)=w2048) -> ()  [unwired: 1 out]
    }
    frame "Oops", Default {
    }
  }
  "Output" <- w9
  "Scan comment" <- w6
